vi "Interfaz grafica.vi"() -> ()   [LabVIEW 2016]
uses:
  Optotune Lens Driver 4 Labview package/Optotune Lens Driver 4 Labview package/Hello Optotune Lens (30.06.2015)/Calibration.ctl
  <vilib>/DAQmx/read.llb/DAQmx Read (Analog 1D Wfm NChan NSamp).vi
  <vilib>/Analysis/2dsp.llb/Decimate (single shot, DBL).vi
  <vilib>/Utility/file.llb/Read Delimited Spreadsheet (string).vi
  <vilib>/DAQmx/miscellaneous.llb/DAQmx Fill In Error Info.vi
  <vilib>/Waveform/WDTOps.llb/WDT Index Channel DBL.vi
  <vilib>/Analysis/2dsp.llb/Decimate (continuous, DBL).vi
  <vilib>/Instr/_visa.llb/VISA Configure Serial Port (Instr).vi
  <vilib>/Utility/file.llb/Write Delimited Spreadsheet (string).vi
  <vilib>/Waveform/WDTOps.llb/WDT Get Waveform Time Array DBL.vi
  <vilib>/Analysis/NI_AALPro.lvlib
panel:
  in  "Restablecer Iniciales":bool
  in  "Incremento":dbl=0.1 format="%#_13g"
  out "Potencia derecho":dbl
  out "error out 4":errorcluster
  out "error out 3":errorcluster
  out "error out 2":errorcluster
  in  "Tab Control 3":enum32{"WL", "Video"}(tab)
  out "Waveform length":dbl[][](graph)
  in  "Escala autom. X":u8=1
  in  "Maximo escala X":dbl
  in  "Minimo escala X":dbl
  in  "Minimo escala Y":dbl format="%#_13g"
  in  "Maximo escala Y":dbl format="%#_13g"
  in  "Escala autom. Y":u8=1
  out "Image Out":T1(plugin-control)
  in  "Carpeta archivo":string="C:\\Users\\TGM1603\\Documents\\LabVIEW Data\\Experimentos electrodos\\VideosExperimentos"
  in  "Modo de video":u16(ring)=21 items=["160x90 I420 30 fps", "160x90 MJPG 30 fps", "160x90 RGB24 30 fps", "160x120 I420 30 fps", "160x120 MJPG 30 fps", "160x120 RGB24 30 fps", "176x144 I420 30 fps", "176x144 MJPG 30 fps", "176x144 RGB24 30 fps", "320x180 I420 30 fps", "320x180 MJPG 30 fps", "320x180 RGB24 30 fps", "320x240  I420 30 fps", "320x240 MJPG 30 fps", "320x240 RGB24 30 fps", "352x288 I420 30 fps", "352x288 MJPG 30 fps", "352x288 RGB24 30 fps", "432x240 I420 30 fps", "432x240 MJPG 30 fps", "432x240 RGB24 30 fps", "640x360 I420 30 fps", "640x360 MJPG 30 fps", "640x360 RGB24 30 fps", "640x480 I420 30 fps", "640x480 MJPG 30 fps", "640x480 RGB24 30 fps", "800x448 I420 30 fps", "800x448 MJPG 30 fps", "800x448 RGB24 30 fps", "800x600 I420 30 fps", "800x600 MJPG 30 fps", "800x600 RGB24 30 fps", "864x480 I420 30 fps", "864x480 MJPG 30 fps", "864x480 RGB24 30 fps", "960x720 I420 30 fps", "960x720 MJPG 30 fps", "960x720 RGB24 30 fps", "1024x576 I420 30 fps", "1024x576 MJPG 30 fps", "1024x576 RGB24 30 fps", "1280x720 I420 30 fps", "1280x720 MJPG 30 fps", "1280x720 RGB24 30 fps", "1600x896 I420 30 fps", "1600x896 MJPG 30 fps", "1600x896 RGB24 30 fps", "1920x1080 I420 5 fps", "1920x1080 MJPG 30 fps", "1920x1080 RGB24 5 fps", "2304x1296 I420 2 fps", "2304x1296 RGB24 2 fps", "2304x1536 I420 2 fps", "2304x1536 RGB24 2 fps"]
  in  "Calidad":u32=1000
  in  "Frame Rate":u32=30
  out "VISA resource name out":string
  in  "Tab Control 2":T2(tab)
  in  "DAQmx Physical Channel":tag
  in  "Frecuencia muestreo":i32=20000
  in  "Rango voltaje":i16(ring)=5 items=["0.1"=0, "1"=1, "5"=5, "10"=10]
  in  "tamaño buffer":i32=1000
  in  "factor decimacion":i32=20
  in  "Ganancia":u16(ring) items=["0.2"=51455, "1"=33023, "10"=49407, "20"=41215, "30"=57599, "40"=37119, "60"=53503, "80"=45311, "120"=61695, "157"=35071, ""=0]
  in  "Potencia inicial lente derecho":dbl(slide) scale=-3.0..3.0
  in  "Potencia inicial lente izquierdo":dbl(slide) scale=-3.0..3.0
  in  "VISA resource name":string="COM11"
  in  "VISA resource name 2":string="COM10"
  out "DPT INICIALES D":dbl
  out "DPT INICIALES I":dbl
  out "Potencia izquierdo":dbl
  in  "error in (no error) 5":errorcluster
  in  "error in (no error) 4":errorcluster
  in  "error in (no error) 3":errorcluster
  in  "error in (no error) 2":errorcluster
  in  "Calibration 4":T3={"Max Current A"=293.0, "Max Current B"=293.0, "UCL A"=300.0, "UCL B"=300.0, "LCL A"=0.0, "LCL B"=0.0} {"Max Current A" format="%#_g mA"; "Max Current B" format="%#_g mA"; "UCL A" format="%#_g mA"; "LCL A" format="%#_g mA"; "UCL B" format="%#_g mA"; "LCL B" format="%#_g mA"}
  out "ID 2":u16
  out "VISA resource name out 2":string
  out "Calibration 3":T3 {"Max Current A" format="%#_g mA"; "Max Current B" format="%#_g mA"; "UCL A" format="%#_g mA"; "LCL A" format="%#_g mA"; "UCL B" format="%#_g mA"; "LCL B" format="%#_g mA"}
  out "OK 2":bool
  out "Data 2":string
  out "Command to Port 2":string
  in  "Cola tipo 2":dbl[](array[numeric])
  out "Distancia":u32
  in  "Tamaño ventana WL":i32=60
  in  "Limite inferior WL":dbl=25.0 format="%#_13g"
  in  "Limite superior WL":dbl=50.0
  out "number":u32
  in  "Calibration":T3={"Max Current A"=293.0, "Max Current B"=293.0, "UCL A"=300.0, "UCL B"=300.0, "LCL A"=0.0, "LCL B"=0.0} {"Max Current A" format="%#_g mA"; "Max Current B" format="%#_g mA"; "UCL A" format="%#_g mA"; "LCL A" format="%#_g mA"; "UCL B" format="%#_g mA"; "LCL B" format="%#_g mA"}
  out "ID":u16
  out "Calibration 2":T3 {"Max Current A" format="%#_g mA"; "Max Current B" format="%#_g mA"; "UCL A" format="%#_g mA"; "LCL A" format="%#_g mA"; "UCL B" format="%#_g mA"; "LCL B" format="%#_g mA"}
  out "OK":bool
  out "Data":string
  out "Command to Port":string
  in  "DPT dif.":dbl
  out "error out":errorcluster
  in  "error in (no error)":errorcluster
  in  "WL":dbl
  in  "Cola tipo":dbl[](array[numeric])
  out "T button?":bool
  in  "Elegir menu Exp":bool
  in  "Elegir menu":bool
  out "path":path
  in  "Iniciar experimento":bool
  in  "Parar adquisicion":bool
  out "Enfermedad visual":string
  out "Edad":string
  out "Nombre":string
  out "Cedula":string
  in  "Carpeta":path=path "C:/Users/TGM1603/Documents/LabVIEW Data/Experimentos electrodos"
  in  "?":bool
  in  "Menu Principal":u16(ring) items=["Visualizacion general ", "Llevar a cabo un experimento", "Ajustar potencia inicial lentes"]
  in  "Menu experimentos":u16(ring) items=["Experimento 1", "Experimento 2", "Experimento 3", "Experimento 4", "", "", "", ""]
  in  "Tab Control":enum32{"Señal EMG", "Potencia y distancia"}(tab)
  out "Senal EMG":waveform(dbl)[](graph)
  in  "Escala automatica Y":u8
  in  "Escala automatica X":u8=1
  in  "X Scale.Range:Increment":dbl
  in  "X Scale.Range:Minimum":dbl
  in  "X Scale.Range:Maximum":dbl
  in  "Y Scale.Range:Minimum":dbl=-5.0
  in  "Y Scale.Range:Maximum":dbl=5.0
  in  "Escala Y min":dbl
  in  "Escala Y max":dbl
  in  "Auto scale Y":u8=1
  in  "Escala X max":dbl
  in  "Escala X min":dbl
  out "Potencia optica y distancia":dbl[][](graph)
  in  "Auto scale X":u8=1
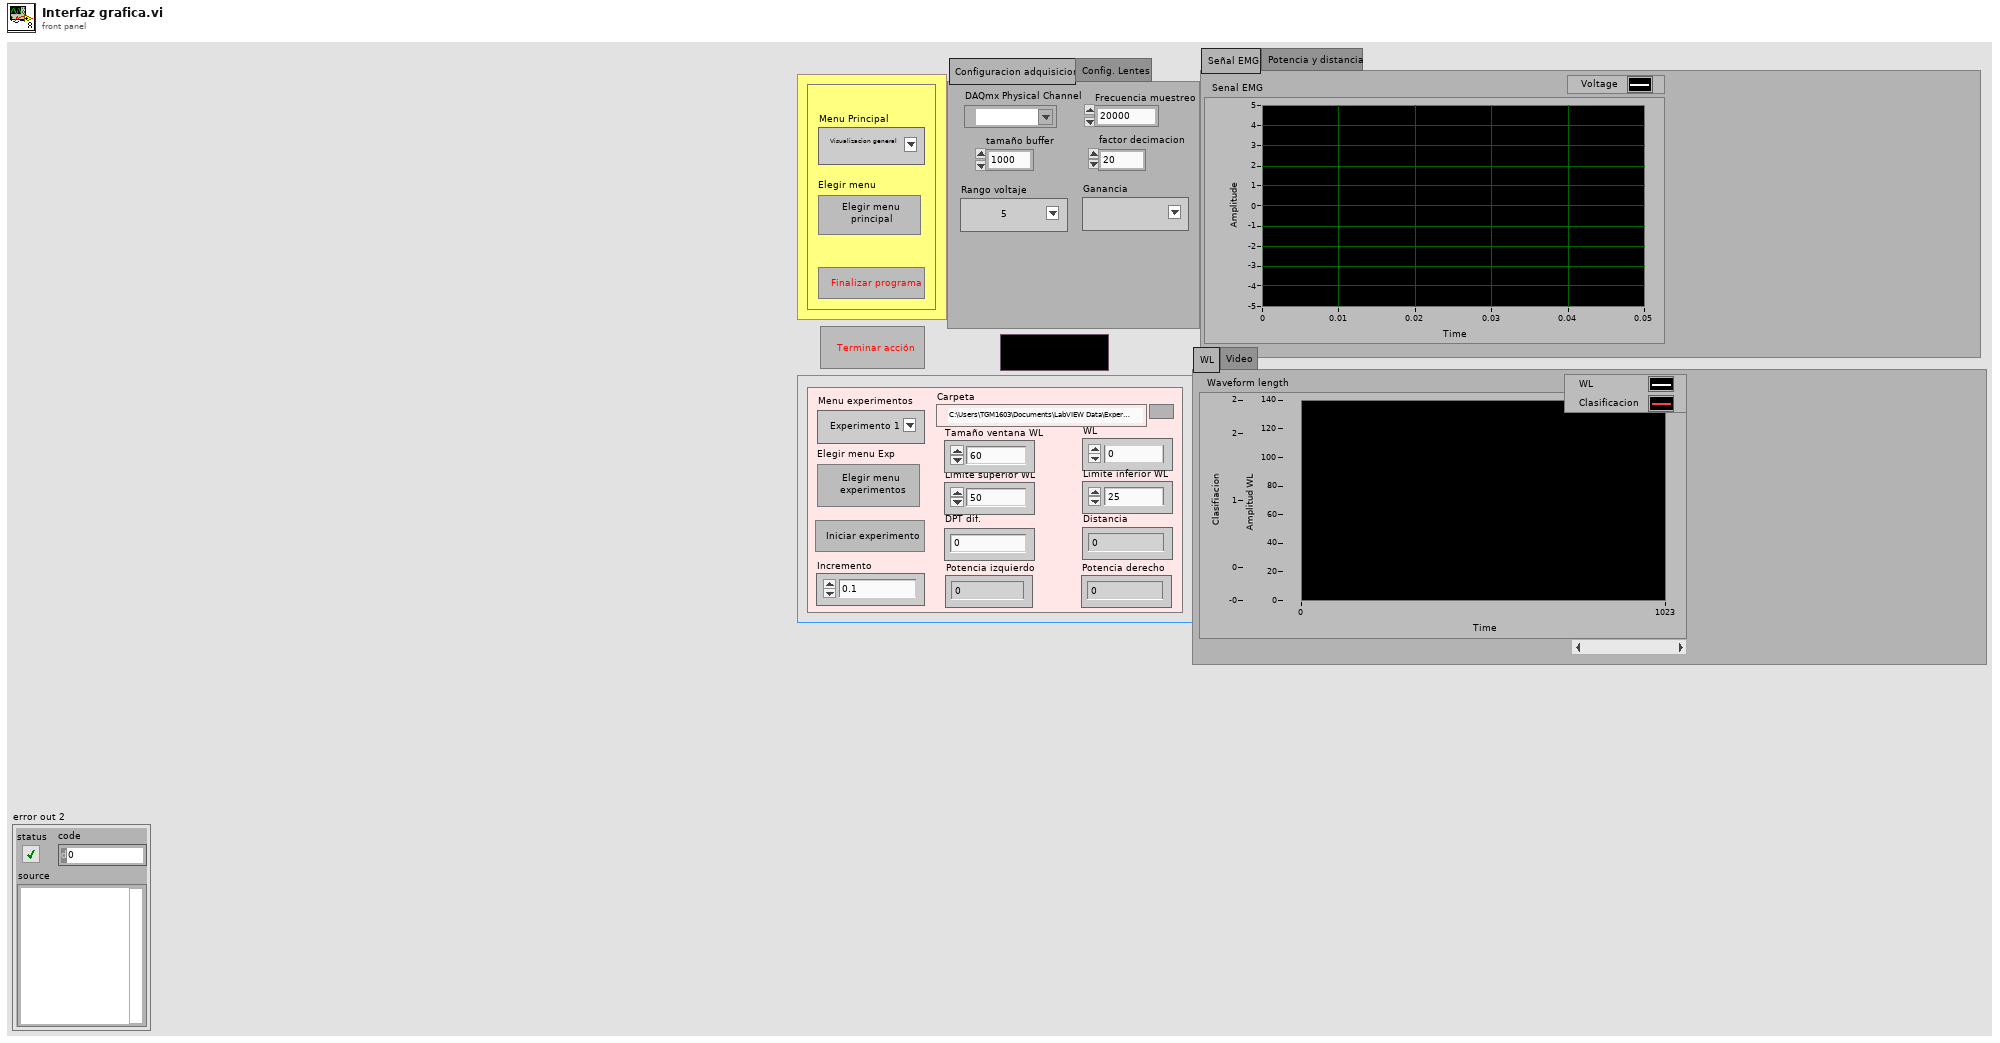
[diagram p1: front panel]
types:
  T1 = typedef "IMAQ Image.ctl" = refnum<image>
  T2 = enum32{"Configuracion adquisicion", "Config. Lentes"}
  T3 = typedef "Calibration.ctl" = cluster{"Max Current A":dbl, "Max Current B":dbl, "UCL A":dbl, "UCL B":dbl, "LCL A":dbl, "LCL B":dbl}
  T4 = enum16{"Left Button", "Center Button", "Right Button", "Window Close"}
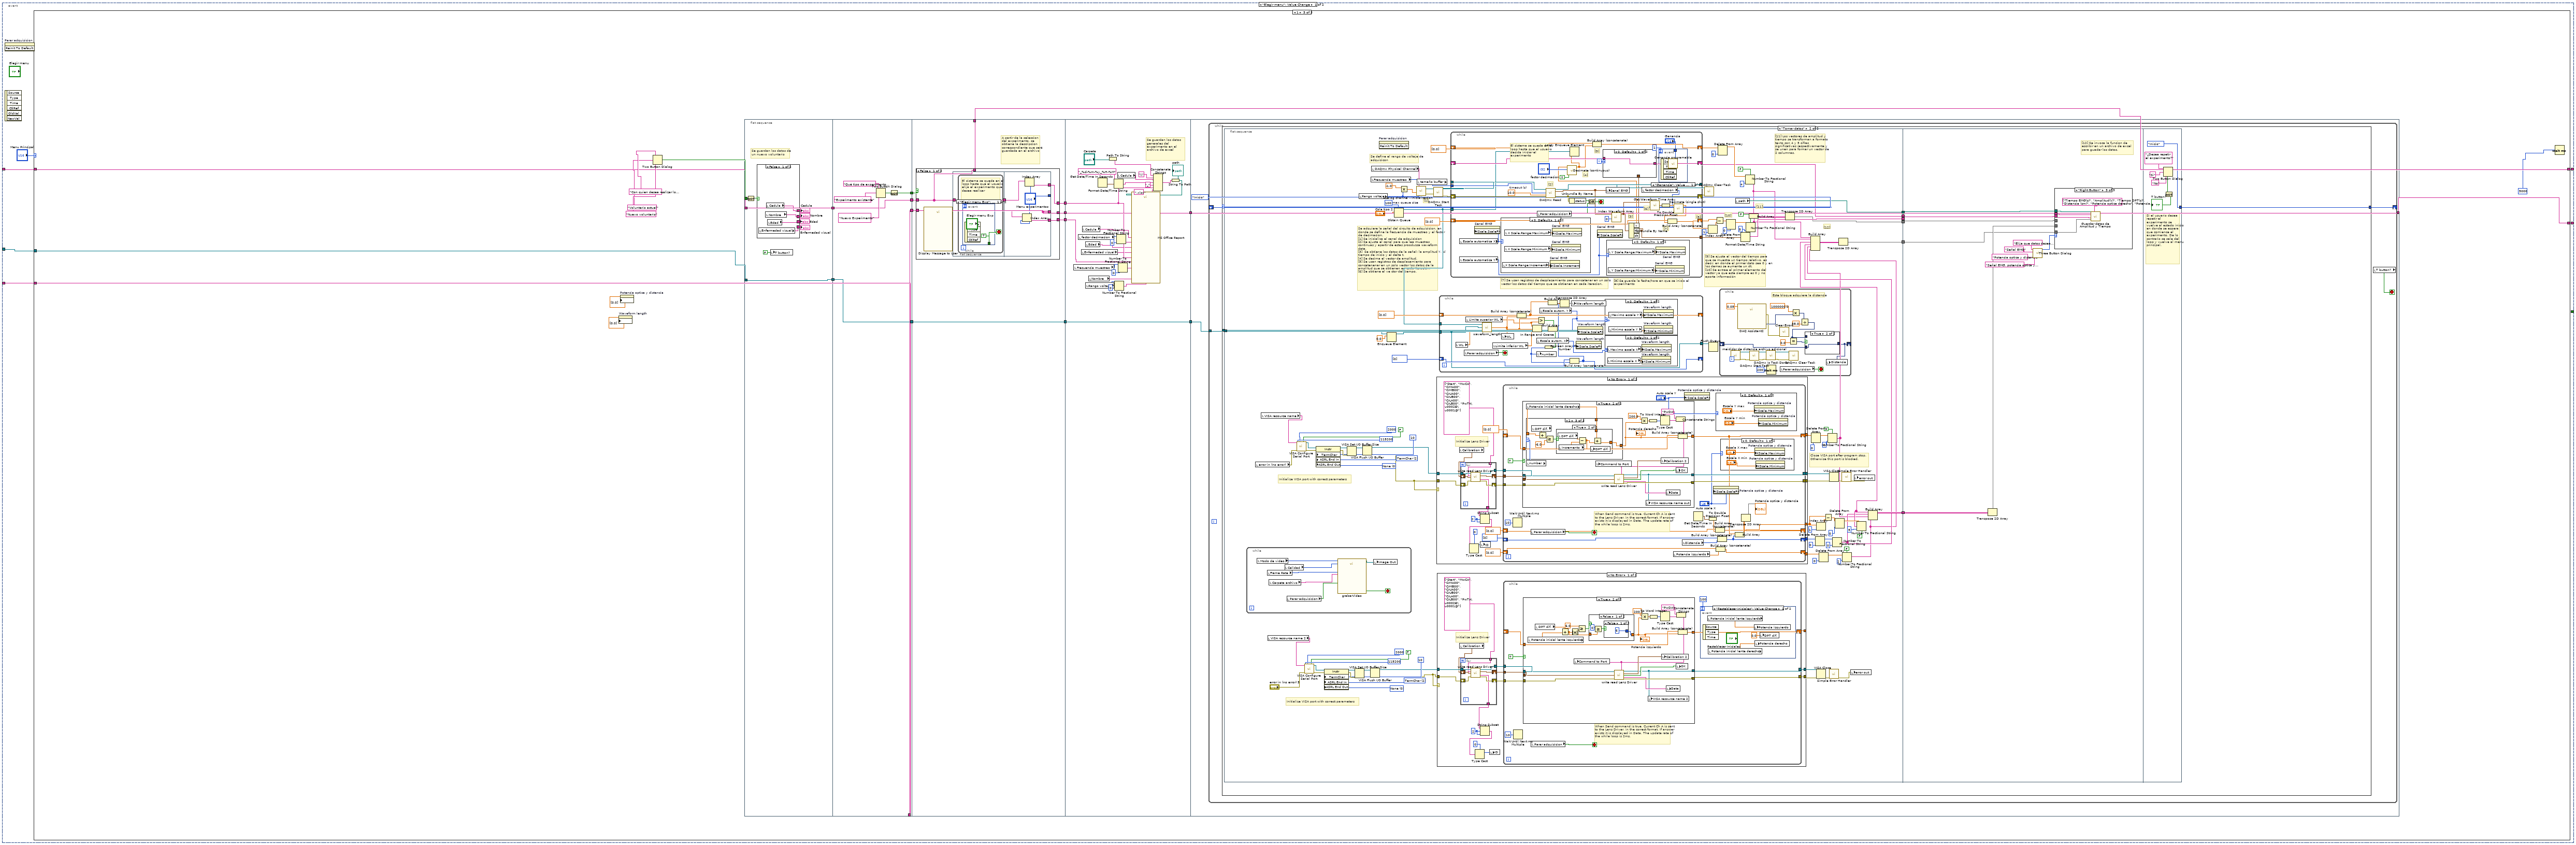
[diagram p2: hidden frame]
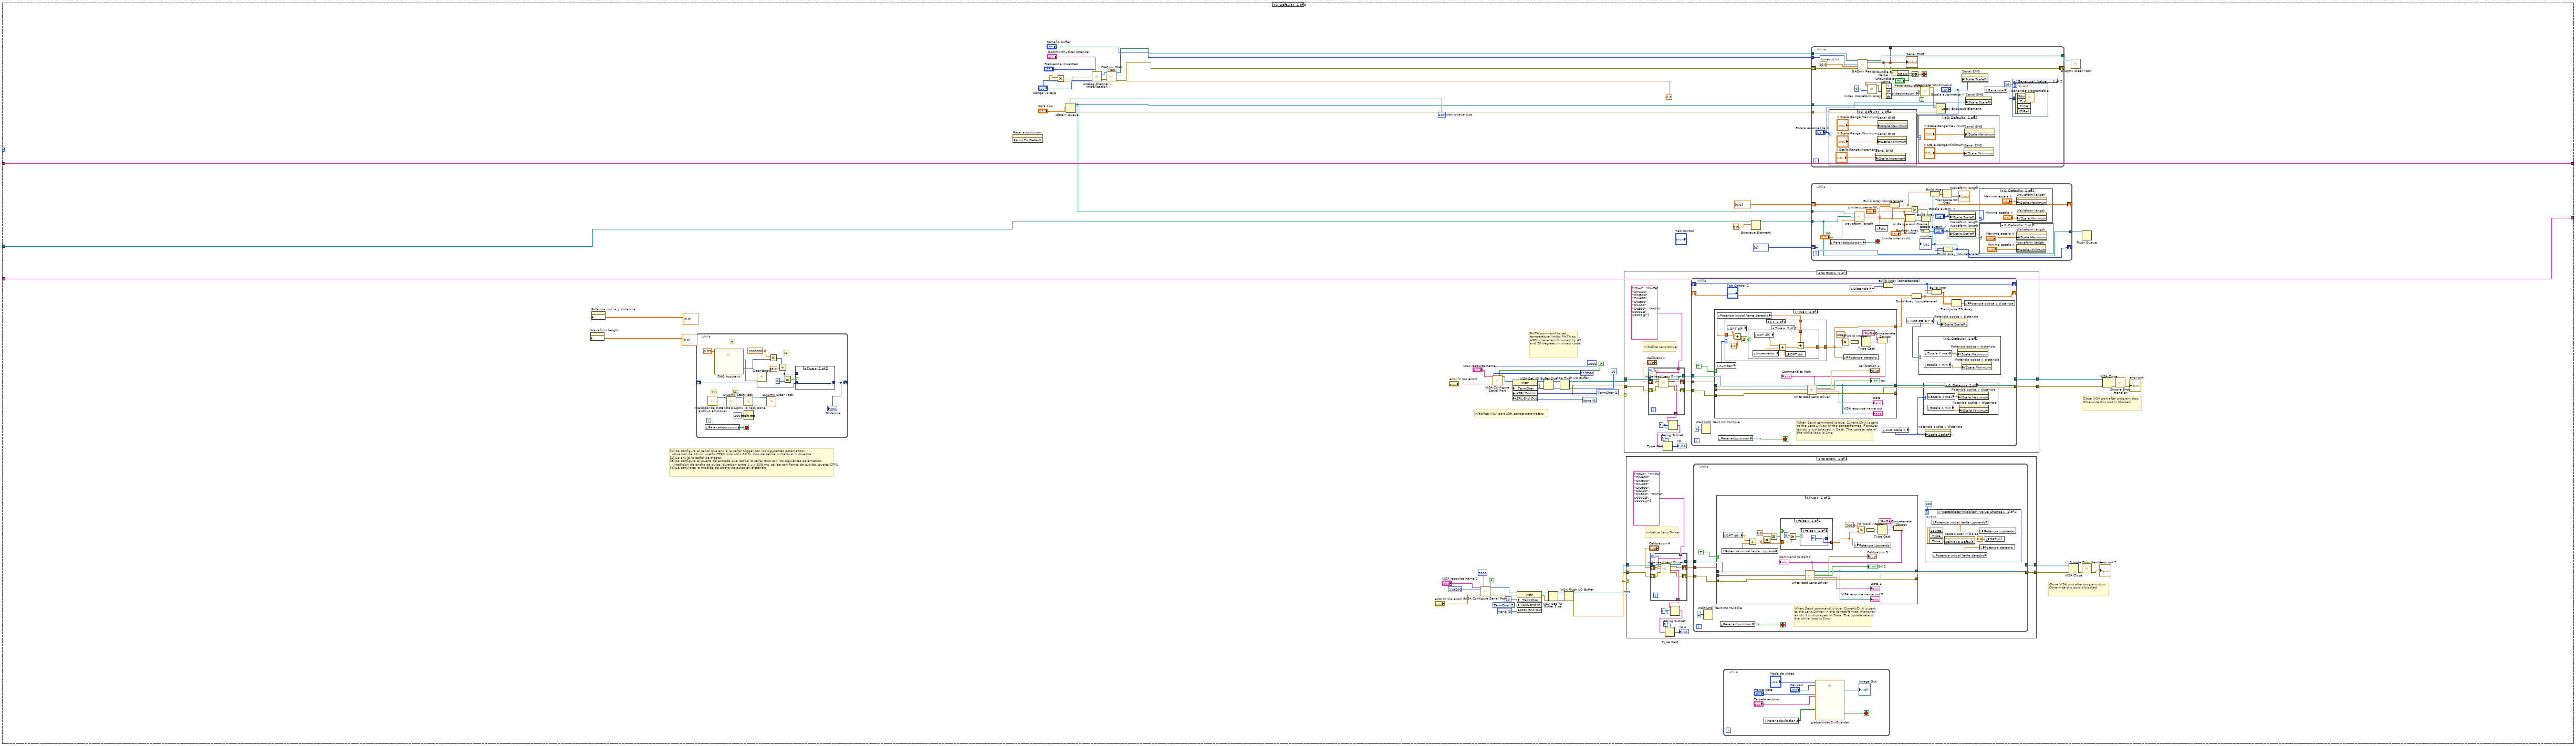
[diagram p3: hidden frame]
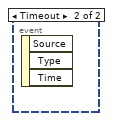
[diagram p4: hidden frame]
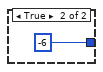
[diagram p6: hidden frame]
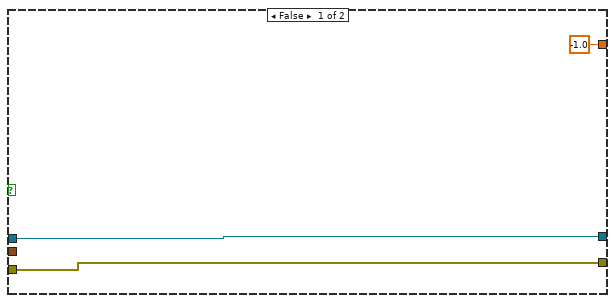
[diagram p12: hidden frame]
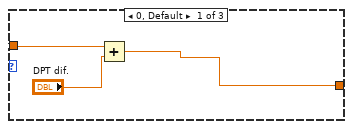
[diagram p13: hidden frame]
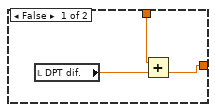
[diagram p14: hidden frame]
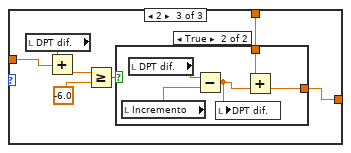
[diagram p15: hidden frame]
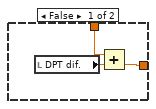
[diagram p16: hidden frame]
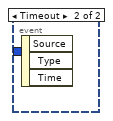
[diagram p20: hidden frame]
diagram:
  # "[1] Se configura el canal que envía la señal trigger con los siguientes parametros:\n  -duracion de 10 us, puerto CTR0,ciclo utilo 50 %, tipo de salida pulsatoria, 1 muestra \n[2] Se envía la señal de trigger.\n[3] Se configura el puerto de entrada que recibe la señal ECO con los siguientes parámetros:\n  - Medicion de ancho de pulso, duracion entre 1 u y 600 ms, se lee con flanco de subida, puerto CTR1\n[4] Se convierte la medida de ancho de pulso en distancia."
  n1 = flat-sequence {
    tunnel: [w18] -> w3
    tunnel: [w15] -> w2
    tunnel: [w10] -> w1
    tunnel: w3 -> [w24]
    tunnel: w2 -> [w23]
    tunnel: w1 -> [w22]
    frame #0 {
      # "Inicializa la cola"
      # "Crea la cola que va a guardar los valores de la sumatoria que calcula el waveform length así como determina la cantidad de valores que se van a sumar(tamaño de la ventana)"
      # "Se obtiene los elementos de la columna 1 que corresponde a  la descripcion de los experimentos"
      # "Se obtiene los elementos de la columna 0 que corresponde al nombre de los experimentos"
      # "Se guarda los experimentos en el menu\n para que el usuario pueda elegir cual \nrealizar"
      # "Se cargan los experimentos  guardados"
      n2 = call-poly <vilib>:"Read Delimited Spreadsheet.vi"("file path (dialog if empty)"=path "C:/Users/TGM1603/Documents/LabVIEW Data/Experimentos_realizados") -> ("all rows"=w19:string[][])  [unwired: 9 in, 5 out]
      n3 = Transpose 2D Array(2D array=w19) -> (transposed array=w16:string[][])
      n4 = Index Array(array=w16, index (row)=1) -> (element=w15:string[])  [unwired: 1 in]
      n5 = Index Array(array=w16, index (row)=0) -> (element=w18:string[])  [unwired: 1 in]
      n6 = property on="Menu experimentos" class="Ring (strict)"("Strings []"=w18) -> ()  [unwired: 2 in, 2 out]
      n7 = Obtain Queue(max queue size (-1, unlimited)="Tamaño ventana WL", element data type=0.0) -> (queue out=w13:refnum<queue>)  [unwired: 3 in, 2 out]
      n8 = property on="Waveform length" class="WFChart (strict)"("History Data"=dbl[][] [[0.0]]) -> ()  [unwired: 2 in, 2 out]
      n9 = property on="Potencia optica y distancia" class="WFChart (strict)"("History Data"=dbl[][] [[0.0]]) -> ()  [unwired: 2 in, 2 out]
      n10 = local write "DPT INICIALES D"(0.0 ("DPT INIT.1")) -> ()
      n11 = local write "DPT INICIALES I"(0.0 ("DPT INIT.2")) -> ()
      n12 = local write "DPT dif."(0.0 ("WL")) -> ()
      n13 = local write "WL"(0.0 ("WL")) -> ()
      n14 = Enqueue Element(queue=w13, element=0.0) -> (queue out=w10:refnum<queue>)  [unwired: 2 in, 2 out]
    }
    frame #1 {
      n15 = while {
        shift-right: [w30] -> _
        shift-left: w24 -> [w31]
        shift-right: [w28] -> _
        shift-left: w23 -> [w29]
        tunnel: w22 -> [w27]
        stop <- w26 stop-if-true
        n16 = event shown="[1] Timeout" {
          selector: _ -> [_ _]
          dyn-events: _ -> [_ _]
          timeout: 10 -> [_ _]
          tunnel: w31 -> [w37 w1048]
          tunnel: [w36 w1048] -> w30
          tunnel: w29 -> [w35 w1047]
          tunnel: [w34 w1047] -> w28
          tunnel: w27 -> [w32 _]
          tunnel: [_ "?"] -> w26
          event "Elegir menu": Value Change {
            n17 = invoke on="Parar adquisicion" class="Bool (strict)" method="Reinit To Default"() -> ()  [unwired: 3 in, 3 out]
            n18 = event-data() -> ()  [unwired: 1 in, 6 out]
            n19 = case shown="1" "Menu Principal" {
              tunnel: w37 -> [w103 w389 w504]
              tunnel: [w103 w389 w503] -> w36
              tunnel: w35 -> [w102 w388 w501]
              tunnel: [w102 w388 w500] -> w34
              tunnel: w32 -> [w85 _ w490]
              frame 0, Default {
                w53 = u16 0 items=["None", "Last Bit", "TermChar", "Break"] ("Serial Settings:End Mode for Writes")
                w52 = u16 2 items=["None", "Last Bit", "TermChar"] ("Serial Settings:End Mode for Reads")
                w75 = u16 0 items=["None", "Last Bit", "TermChar", "Break"] ("Serial Settings:End Mode for Writes")
                w76 = u16 2 items=["None", "Last Bit", "TermChar"] ("Serial Settings:End Mode for Reads")
                w89 = 100  # max queue size
                # "Close VISA port after program stop. Otherwise this port is blocked."
                # "[1] Se configura el canal que envía la señal trigger con los siguientes parametros:\n  -duracion de 10 us, puerto CTR0,ciclo utilo 50 %, tipo de salida pulsatoria, 1 muestra \n[2] Se envía la señal de trigger.\n[3] Se configura el puerto de entrada que recibe la señal ECO con los siguientes parámetros:\n  - Medicion de ancho de pulso, duracion entre 1 u y 600 ms, se lee con flanco de subida, puerto CTR1\n[4] Se convierte la medida de ancho de pulso en distancia."
                # "PwTA command to set temperature limits: PwTA as ASCII characters followed by 45 and 20 degrees in binary code."
                # "Close VISA port after program stop. Otherwise this port is blocked."
                # "Initialize VISA port with correct parameters"
                n20 = property on="Waveform length" class="WFChart (strict)"("History Data"=dbl[][] [[0.0]]) -> ()  [unwired: 2 in, 2 out]
                n21 = property on="Potencia optica y distancia" class="WFChart (strict)"("History Data"=dbl[][] [[0.0]]) -> ()  [unwired: 2 in, 2 out]
                n22 = while {
                  shift-right: [w178] -> _
                  shift-left: _ -> [w177]
                  stop <- w182 stop-if-true
                  # "[4]"
                  # "[3]"
                  # "[2]"
                  # "[1]"
                  n23 = local read "Parar adquisicion"() -> (w182:bool)
                  n24 = call "meididor de distancia archivo adicional.vi"() -> ("error out"=w185:errorcluster, "task out"=w186:refnum<k21>)  [unwired: 10 in]
                  n25 = call "DAQ Assistant"("timeout (s)"=0.05) -> ("data"=w195:dynamicdata, "error out"=w183:errorcluster)  [unwired: 16 in, 1 out]
                  n26 = call <vilib>:"DAQmx Start Task.vi"("task/channels in"=w186, "error in"=w185) -> ("task out"=w189:refnum<k21>, "error out"=w190:errorcluster)  [unwired: 12 in]
                  n27 = call <vilib>:"DAQmx Is Task Done.vi"("task/channels in"=w189, "error in"=w190) -> ("task out"=w187:refnum<k21>, "error out"=w188:errorcluster)  [unwired: 11 in, 1 out]
                  n28 = Wait (ms)(milliseconds to wait=u32 200) -> ()  [unwired: 1 out]
                  n29 = call <vilib>:"Clear Errors.vi"("error in (no error)"=w183) -> ()  [unwired: 5 in, 2 out]
                  n30 = call <vilib>:"DAQmx Clear Task.vi"("task in"=w187, "error in"=w188) -> ()  [unwired: 13 in, 1 out]
                  n31 = Multiply(x=1000000.0, y=w195) -> (x*y=w193:dynamicdata)
                  n32 = Divide(x=w193, y=58.0) -> (x/y=w179:dynamicdata)
                  n33 = Equal?(x=w179, y=u16 0) -> (x = y?=w181:dynamicdata)
                  n34 = case shown="True" w181 {
                    tunnel: [w196 w197] -> w178
                    tunnel: w179 -> [w196 _]
                    tunnel: w177 -> [_ w197]
                    frame False {
                    }
                    frame True {
                    }
                  }
                  "Distancia" <- w178
                }
                n35 = invoke on="Parar adquisicion" class="Bool (strict)" method="Reinit To Default"() -> ()  [unwired: 3 in, 3 out]
                n36 = Multiply(x=-1.0 ("y"), y="Rango voltaje") -> (x*y=w92:dbl)
                n37 = Obtain Queue(max queue size (-1, unlimited)=w89, element data type="Cola tipo") -> (queue out=w86:refnum<queue>, error out=w87:errorcluster)  [unwired: 3 in, 1 out]
                n38 = call "Analog channel - inicializacion.vi"("maximum value"="Rango voltaje", "minimum value"=w92, "rate"="Frecuencia muestreo", "DAQmx Physical Channel"="DAQmx Physical Channel") -> ("error out"=w95:errorcluster, "task out"=w96:refnum<k21>)
                n39 = call <vilib>:"DAQmx Start Task.vi"("task/channels in"=w96, "error in"=w95) -> ("task out"=w101:refnum<k21>, "error out"=w100:errorcluster)  [unwired: 12 in]
                n40 = call-poly "VISA Configure Serial Port"("VISA resource name"="VISA resource name 2", "timeout (10sec)"=u32 2000, "Enable Termination\nChar (T)"=FALSE ("Enable Termination\nChar (T)"), "baud rate (9600)"=u32 115200, "error in (no error)"="error in (no error) 2") -> ("VISA resource name out"=w48:refnum<visa-resource-name>, "error out"=w50:errorcluster)  [unwired: 9 in]
                n41 = call-poly "VISA Configure Serial Port"("VISA resource name"="VISA resource name", "timeout (10sec)"=u32 2000, "Enable Termination\nChar (T)"=FALSE ("Enable Termination\nChar (T)"), "baud rate (9600)"=u32 115200, "error in (no error)"="error in (no error)") -> ("VISA resource name out"=w80:refnum<visa-resource-name>, "error out"=w78:errorcluster)  [unwired: 9 in]
                n42 = property class="Instr"(reference=w80, error in=w78, "TermChar"=u8 10 ("Message Based Settings:Termination Character"), "ASRL End In"=w76, "ASRL End Out"=w75) -> (reference out=w79:refnum<visa-resource-name>, error out=w77:errorcluster)
                n43 = property class="Instr"(reference=w48, error in=w50, "TermChar"=u8 10 ("Message Based Settings:Termination Character"), "ASRL End In"=w52, "ASRL End Out"=w53) -> (reference out=w49:refnum<visa-resource-name>, error out=w51:errorcluster)
                n44 = VISA Set I/O Buffer Size(VISA resource name=w79, error in (no error)=w77) -> (VISA resource name out=w72:refnum<visa-resource-name>, error out=w71:errorcluster)  [unwired: 2 in]
                n45 = VISA Set I/O Buffer Size(VISA resource name=w49, error in (no error)=w51) -> (VISA resource name out=w56:refnum<visa-resource-name>, error out=w57:errorcluster)  [unwired: 2 in]
                n46 = VISA Flush I/O Buffer(VISA resource name=w72, error in (no error)=w71) -> (VISA resource name out=w70:refnum<visa-resource-name>, error out=w65:errorcluster)  [unwired: 1 in]
                n47 = VISA Flush I/O Buffer(VISA resource name=w56, error in (no error)=w57) -> (VISA resource name out=w42:refnum<visa-resource-name>, error out=w43:errorcluster)  [unwired: 1 in]
                n48 = case shown="No Error" w65 {
                  tunnel: w65 -> [w211 w295]
                  tunnel: w70 -> [w210 w296]
                  tunnel: [w209 w295] -> w68
                  tunnel: [w208 w296] -> w66
                  frame No Error {
                    w206 = 2 ("length (rest)")
                    # "Initialize Lens Driver"
                    n49 = for {
                      tunnel: w210 -> [w293]
                      tunnel: [w290] -> w200
                      tunnel: string[] ["Start", "MwCA", "CrMA00", "CrMB00", "CrUA00", "CrUB00", "CrLA00", "CrLB00", "PwTA\u0002Ð\u0001@"] -> [w288] mode=indexing
                      tunnel: [w287] -> w199
                      shift-right: [w291] -> w201
                      shift-left: "Calibration" -> [w292]
                      shift-right: [w289] -> w202
                      shift-left: w211 -> [w294]
                      n50 = call "write read Lens Driver.vi"("VISA resource name"=w293, "command"=w288, "Calibration"=w292, "error in (no error)"=w294) -> ("VISA resource name out"=w290:refnum<visa-resource-name>, "Calibration 2"=w291:T3, "Data"=w287:string, "error out"=w289:errorcluster)  [unwired: 4 in, 4 out]
                    }
                    n51 = String Subset(string=w199, offset (0)=w206, length (rest)=w206) -> (substring=w204:string)
                    n52 = Type Cast(type=u16 0 ("length (rest)"), x=w204) -> (*(type *) &x=→"ID":u16)
                    n53 = while {
                      tunnel: [w223] -> w209
                      tunnel: [w224] -> w208
                      tunnel: w202 -> [w229]
                      tunnel: w201 -> [w228]
                      tunnel: w200 -> [w227]
                      shift-right: [w214] -> _
                      shift-left: _ -> [w218]
                      shift-right: [w215] -> _
                      shift-left: _ -> [w217]
                      stop <- w222 stop-if-true
                      # "When Send command is true, Current Ch A is sent to the Lens Driver, in the correct format. If answer exists it is displayed in Data. The update rate of the while loop is 2ms."
                      n54 = Wait Until Next ms Multiple(millisecond multiple=u32 2) -> ()  [unwired: 1 out]
                      n55 = case shown="True" TRUE ("Send command") {
                        tunnel: [w236 w253] -> w223
                        tunnel: w229 -> [w236 w252]
                        tunnel: w228 -> [_ w246]
                        tunnel: w227 -> [w235 w251]
                        tunnel: [w235 w248] -> w224
                        tunnel: [-1.0 ("DPT") w237] -> w216
                        frame False {
                        }
                        frame True {
                          n56 = local read "number"() -> (w239:u32)
                          n57 = local read "Potencia inicial lente derecho"() -> (w238:dbl)
                          n58 = case shown="1" w239 {
                            tunnel: [w255 w263 w278] -> w237
                            tunnel: w238 -> [w256 w258 w273]
                            tunnel: w238 -> [_ w257 w272]
                            frame 0, Default {
                              n59 = Add(x=w256, y="DPT dif.") -> (x+y=w255:dbl)
                            }
                            frame 1 {
                              n60 = local read "DPT dif."() -> (w259:dbl)
                              n61 = Add(x=w258, y=w259) -> (x+y=w260:dbl)
                              n62 = Less Or Equal?(x=w260, y=6.0) -> (x <= y?=w262:bool)
                              n63 = case shown="True" w262 {
                                tunnel: [w265 w269] -> w263
                                tunnel: w257 -> [w264 w268]
                                frame False {
                                n64 = local read "DPT dif."() -> (w266:dbl)
                                n65 = Add(x=w264, y=w266) -> (x+y=w265:dbl)
                                }
                                frame True {
                                n66 = local read "Incremento"() -> (w267:dbl)
                                n67 = local read "DPT dif."() -> (w270:dbl)
                                n68 = Add(x=w270, y=w267) -> (x+y=w271:dbl)
                                n69 = local write "DPT dif."(w271) -> ()
                                n70 = Add(x=w268, y=w271) -> (x+y=w269:dbl)
                                }
                              }
                            }
                            frame 2 {
                              n71 = local read "DPT dif."() -> (w277:dbl)
                              n72 = Add(x=w277, y=w273) -> (x+y=w274:dbl)
                              n73 = Greater Or Equal?(x=w274, y=-6.0) -> (x >= y?=w275:bool)
                              n74 = case shown="True" w275 {
                                tunnel: [w280 w284] -> w278
                                tunnel: w272 -> [w279 w283]
                                frame False {
                                n75 = local read "DPT dif."() -> (w281:dbl)
                                n76 = Add(x=w279, y=w281) -> (x+y=w280:dbl)
                                }
                                frame True {
                                n77 = local read "Incremento"() -> (w282:dbl)
                                n78 = local read "DPT dif."() -> (w286:dbl)
                                n79 = Subtract(x=w286, y=w282) -> (x-y=w285:dbl)
                                n80 = local write "DPT dif."(w285) -> ()
                                n81 = Add(x=w283, y=w285) -> (x+y=w284:dbl)
                                }
                              }
                            }
                          }
                          n82 = Multiply(x=200.0, y=w237) -> (x*y=w244:dbl)
                          n83 = local write "Potencia derecho"(w237) -> ()
                          n84 = To Word Integer(number=w244) -> (16bit integer=w243:i16)
                          n85 = Type Cast(x=w243) -> (*(type *) &x=w242:string)  [unwired: 1 in]
                          n86 = Concatenate Strings("PwDA", w242) -> (w240:string)
                          "Command to Port" <- w240
                          n87 = call "write read Lens Driver.vi"("VISA resource name"=w251, "command"=w240, "Calibration"=w246, "error in (no error)"=w252) -> ("VISA resource name out"=w248:refnum<visa-resource-name>, "Calibration 2"=→"Calibration 2":T3, "OK"=→"OK":bool, "Data"=→"Data":string, "error out"=w253:errorcluster)  [unwired: 4 in, 3 out]
                          "VISA resource name out" <- w248
                        }
                      }
                      n88 = local read "Parar adquisicion"() -> (w222:bool)
                      n89 = local read "Distancia"() -> (w219:u32)
                      n90 = local read "Auto scale X"() -> (w220:u8)
                      n91 = Build Array (concatenate)(w218, w219) -> (w214:u32[])
                      n92 = local read "Auto scale Y"() -> (w221:u8)
                      n93 = Build Array (concatenate)(w217, w216) -> (w215:dbl[])
                      n94 = case shown="0, Default" w221 {
                        frame 0, Default {
                          n95 = local read "Escala Y min"() -> (w232:dbl)
                          n96 = local read "Escala Y max"() -> (w233:dbl)
                          n97 = property on="Potencia optica y distancia" class="WFChart (strict)"("YScale.Maximum"=w233) -> ()  [unwired: 2 in, 2 out]
                          n98 = property on="Potencia optica y distancia" class="WFChart (strict)"("YScale.Minimum"=w232) -> ()  [unwired: 2 in, 2 out]
                        }
                        frame 1 {
                        }
                      }
                      n99 = case shown="0, Default" w220 {
                        frame 0, Default {
                          n100 = local read "Escala X min"() -> (w230:dbl)
                          n101 = local read "Escala X max"() -> (w231:dbl)
                          n102 = property on="Potencia optica y distancia" class="WFChart (strict)"("XScale.Maximum"=w231) -> ()  [unwired: 2 in, 2 out]
                          n103 = property on="Potencia optica y distancia" class="WFChart (strict)"("XScale.Minimum"=w230) -> ()  [unwired: 2 in, 2 out]
                        }
                        frame 1 {
                        }
                      }
                      n104 = property on="Potencia optica y distancia" class="WFChart (strict)"("XScale.ScaleFit"=w220) -> ()  [unwired: 2 in, 2 out]
                      n105 = Build Array(w215, w214) -> (w213:dbl[][])
                      n106 = property on="Potencia optica y distancia" class="WFChart (strict)"("YScale.ScaleFit"=w221) -> ()  [unwired: 2 in, 2 out]
                      n107 = Transpose 2D Array(2D array=w213) -> (transposed array=w212:dbl[][])
                      n108 = local write "Potencia optica y distancia"(w212) -> ()
                    }
                  }
                  frame Error {
                  }
                }
                n109 = case shown="No Error" w43 {
                  tunnel: w43 -> [w124 w175]
                  tunnel: w42 -> [w123 w176]
                  tunnel: [w122 w175] -> w38
                  tunnel: [w121 w176] -> w39
                  frame No Error {
                    w119 = 2 ("length (rest)")
                    # "Initialize Lens Driver"
                    n110 = for {
                      tunnel: w123 -> [w173]
                      tunnel: [w170] -> w113
                      tunnel: string[] ["Start", "MwCA", "CrMA00", "CrMB00", "CrUA00", "CrUB00", "CrLA00", "CrLB00", "PwTA\u0002Ð\u0001@"] -> [w168] mode=indexing
                      tunnel: [w167] -> w112
                      shift-right: [w171] -> w114
                      shift-left: "Calibration 4" -> [w172]
                      shift-right: [w169] -> w115
                      shift-left: w124 -> [w174]
                      n111 = call "write read Lens Driver.vi"("VISA resource name"=w173, "command"=w168, "Calibration"=w172, "error in (no error)"=w174) -> ("VISA resource name out"=w170:refnum<visa-resource-name>, "Calibration 2"=w171:T3, "Data"=w167:string, "error out"=w169:errorcluster)  [unwired: 4 in, 4 out]
                    }
                    n112 = String Subset(string=w112, offset (0)=w119, length (rest)=w119) -> (substring=w117:string)
                    n113 = Type Cast(type=u16 0 ("length (rest)"), x=w117) -> (*(type *) &x=→"ID 2":u16)
                    n114 = while {
                      tunnel: [w127] -> w122
                      tunnel: [w128] -> w121
                      tunnel: w115 -> [w133]
                      tunnel: w114 -> [w132]
                      tunnel: w113 -> [w131]
                      stop <- w126 stop-if-true
                      # "When Send command is true, Current Ch A is sent to the Lens Driver, in the correct format. If answer exists it is displayed in Data. The update rate of the while loop is 2ms."
                      n115 = Wait Until Next ms Multiple(millisecond multiple=u32 2) -> ()  [unwired: 1 out]
                      n116 = case shown="True" TRUE ("Send command") {
                        tunnel: [w138 w159] -> w127
                        tunnel: w133 -> [w138 w158]
                        tunnel: w132 -> [_ w152]
                        tunnel: w131 -> [w137 w157]
                        tunnel: [w137 w154] -> w128
                        frame False {
                        }
                        frame True {
                          n117 = local read "Potencia inicial lente izquierdo"() -> (w144:dbl)
                          n118 = local read "DPT dif."() -> (w145:dbl)
                          n119 = Add(x=w145, y=w144) -> (x+y=w140:dbl)
                          n120 = Absolute Value(x=w140) -> (abs(x)=w142:dbl)
                          n121 = Greater Or Equal?(x=6.0, y=w142) -> (x >= y?=w143:bool)
                          n122 = case shown="False" w143 {
                            tunnel: w140 -> [w162 w166]
                            tunnel: [w160 w166] -> w139
                            frame False {
                              n123 = Greater Or Equal?(x=u16 0, y=w162) -> (x >= y?=w163:bool)
                              n124 = case shown="False" w163 {
                                tunnel: [i16 6 ("x") i16 -6 ("x")] -> w160
                                frame False {
                                }
                                frame True {
                                }
                              }
                            }
                            frame True {
                            }
                          }
                          n125 = local write "Potencia izquierdo"(w139) -> ()
                          n126 = Multiply(x=200.0, y=w139) -> (x*y=w150:dbl)
                          n127 = To Word Integer(number=w150) -> (16bit integer=w149:i16)
                          n128 = Type Cast(x=w149) -> (*(type *) &x=w148:string)  [unwired: 1 in]
                          n129 = Concatenate Strings("PwDA", w148) -> (w146:string)
                          "Command to Port 2" <- w146
                          n130 = call "write read Lens Driver.vi"("VISA resource name"=w157, "command"=w146, "Calibration"=w152, "error in (no error)"=w158) -> ("VISA resource name out"=w154:refnum<visa-resource-name>, "Calibration 2"=→"Calibration 3":T3, "OK"=→"OK 2":bool, "Data"=→"Data 2":string, "error out"=w159:errorcluster)  [unwired: 4 in, 3 out]
                          "VISA resource name out 2" <- w154
                        }
                      }
                      n131 = local read "Parar adquisicion"() -> (w126:bool)
                      n132 = event shown="[0] \"Restablecer Iniciales\": Value Change" {
                        selector: _ -> [_ _]
                        dyn-events: _ -> [_ _]
                        timeout: 100 -> [_ _]
                        event "Restablecer Iniciales": Value Change {
                          n133 = event-data() -> ()  [unwired: 1 in, 3 out]
                          n134 = local read "Potencia inicial lente izquierdo"() -> (w134:dbl)
                          n135 = local read "Potencia inicial lente derecho"() -> (w135:dbl)
                          n136 = invoke on="Restablecer Iniciales" class="Bool" method="Reinit To Default"() -> ()  [unwired: 3 in, 3 out]
                          n137 = local write "Potencia izquierdo"(w134) -> ()
                          n138 = local write "Potencia derecho"(w135) -> ()
                          n139 = local write "DPT dif."(0.0 ("DPT dif.")) -> ()
                        }
                        event Timeout {
                          n140 = event-data() -> ()  [unwired: 1 in, 3 out]
                        }
                      }
                    }
                  }
                  frame Error {
                  }
                }
                n141 = while {
                  stop <- w109 stop-if-true
                  n142 = local read "Parar adquisicion"() -> (w104:bool)
                  n143 = call "grabarVideoSinGuardar.vi"("VideoMode"="Modo de video", "Quality"="Calidad", "Stop (F)"=w104, "Image Logging Path"="Carpeta archivo", "Frame Rate"="Frame Rate") -> ("Image Out"=→"Image Out":T1, "Stopped"=w109:bool)  [unwired: 20 in, 1 out]
                }
                n144 = Enqueue Element(queue=w85, element=0.0) -> (queue out=w62:refnum<queue>)  [unwired: 2 in, 2 out]
                n145 = while {
                  tunnel: w62 -> [w298]
                  tunnel: w86 -> [w315]
                  shift-right: [w301] -> _
                  shift-left: dbl[] [0.0] -> [w312]
                  shift-right: [w300] -> _
                  shift-left: u32[] [0] -> [w302]
                  tunnel: [w298] -> w60
                  stop <- w313 stop-if-true
                  n146 = local read "Parar adquisicion"() -> (w313:bool)
                  n147 = call "waveform_length.vi"("WL"="WL", "Cola WL"=w298, "Datos entrada"=w315) -> ("WL 2"=w310:dbl)
                  n148 = local write "WL"(w310) -> ()
                  n149 = Build Array (concatenate)(w312, w310) -> (w301:dbl[])
                  n150 = In Range and Coerce(upper limit="Limite superior WL", x=w310, lower limit="Limite inferior WL") -> (In Range?=w308:bool)  [unwired: 1 out]
                  n151 = Greater?(x=w310, y="Limite superior WL") -> (0:w309:bool)
                  n152 = Build Array(w309, w308) -> (w307:bool[])
                  n153 = Boolean Array To Number(Boolean array=w307) -> (number=w303:u32)
                  "number" <- w303
                  n154 = Build Array (concatenate)(w302, w303) -> (w300:u32[])
                  n155 = Build Array(w301, w300) -> (w299:dbl[][])
                  n156 = Transpose 2D Array(2D array=w299) -> (transposed array=→"Waveform length":dbl[][])
                  n157 = property on="Waveform length" class="WFChart (strict)"("YScale.ScaleFit"="Escala autom. Y") -> ()  [unwired: 2 in, 2 out]
                  n158 = property on="Waveform length" class="WFChart (strict)"("XScale.ScaleFit"="Escala autom. X") -> ()  [unwired: 2 in, 2 out]
                  n159 = case shown="0, Default" "Escala autom. Y" {
                    frame 0, Default {
                      n160 = property on="Waveform length" class="WFChart (strict)"("YScale.Maximum"="Maximo escala Y") -> ()  [unwired: 2 in, 2 out]
                      n161 = property on="Waveform length" class="WFChart (strict)"("YScale.Minimum"="Minimo escala Y") -> ()  [unwired: 2 in, 2 out]
                    }
                    frame 1 {
                    }
                  }
                  n162 = case shown="0, Default" "Escala autom. X" {
                    frame 0, Default {
                      n163 = property on="Waveform length" class="WFChart (strict)"("XScale.Maximum"="Maximo escala X") -> ()  [unwired: 2 in, 2 out]
                      n164 = property on="Waveform length" class="WFChart (strict)"("XScale.Minimum"="Minimo escala X") -> ()  [unwired: 2 in, 2 out]
                    }
                    frame 1 {
                    }
                  }
                }
                n165 = while {
                  tunnel: w101 -> [w341]
                  tunnel: "tamaño buffer" -> [w338]
                  tunnel: [w339] -> w97
                  shift-right: [w336] -> w98
                  shift-left: w100 -> [w340]
                  tunnel: [w330] -> _
                  tunnel: w86 -> [w326]
                  tunnel: w87 -> [w325]
                  stop <- w335 stop-if-true
                  w334 = 10.0  # timeout (s)
                  n166 = case shown="0, Default" "Escala automatica X" {
                    frame 0, Default {
                      n167 = property on="Senal EMG" class="WFGraph (strict)"("XScale.Increment"="X Scale.Range:Increment") -> ()  [unwired: 2 in, 2 out]
                      n168 = property on="Senal EMG" class="WFGraph (strict)"("XScale.Minimum"="X Scale.Range:Minimum") -> ()  [unwired: 2 in, 2 out]
                      n169 = property on="Senal EMG" class="WFGraph (strict)"("XScale.Maximum"="X Scale.Range:Maximum") -> ()  [unwired: 2 in, 2 out]
                    }
                    frame 1 {
                    }
                  }
                  n170 = call-poly <vilib>:"DAQmx Read.vi"("task/channels in"=w341, "number of samples per channel"=w338, "timeout"=w334, "error in"=w340) -> ("task out"=w339:refnum<k21>, "data"=w330:waveform(dbl)[], "error out"=w336:errorcluster)  [unwired: 9 in]
                  "Senal EMG" <- w330
                  n171 = call-poly <vilib>:"Index Waveform Array.vi"("index"=0, "waveform array"=w330) -> ("waveform"=w331:waveform(dbl))  [unwired: 8 in, 1 out]
                  n172 = Unbundle By Name(w331) -> ("Y"=w328:dbl[])  [unwired: 2 out]
                  n173 = local read "factor decimacion"() -> (w327:i32)
                  n174 = Unbundle By Name(w336) -> ("status"=w337:bool)
                  n175 = Or(x=w337, y="Parar adquisicion") -> (x .or. y?=w335:bool)
                  n176 = case shown="0, Default" "Escala automatica Y" {
                    frame 0, Default {
                      n177 = property on="Senal EMG" class="WFGraph (strict)"("YScale.Minimum"="Y Scale.Range:Minimum") -> ()  [unwired: 2 in, 2 out]
                      n178 = property on="Senal EMG" class="WFGraph (strict)"("YScale.Maximum"="Y Scale.Range:Maximum") -> ()  [unwired: 2 in, 2 out]
                    }
                    frame 1 {
                    }
                  }
                  n179 = call-poly <vilib>:"Decimate (continuous).vi"("averaging"=TRUE, "decimating factor"=w327, "X"=w328) -> ("Decimated Array"=w324:dbl[])  [unwired: 7 in, 1 out]
                  n180 = Lossy Enqueue Element(queue=w326, element=w324, error in (no error)=w325) -> ()  [unwired: 4 out]
                  n181 = property on="Senal EMG" class="WFGraph (strict)"("YScale.ScaleFit"="Escala automatica Y") -> ()  [unwired: 2 in, 2 out]
                  n182 = property on="Senal EMG" class="WFGraph (strict)"("XScale.ScaleFit"="Escala automatica X") -> ()  [unwired: 2 in, 2 out]
                  n183 = local read "Ganancia"() -> (w321:u16)
                  n184 = event shown="[0] \"Ganancia\": Value Change" {
                    selector: _ -> [_ _]
                    dyn-events: _ -> [_ _]
                    timeout: 10 -> [_ _]
                    tunnel: w321 -> [w342 _]
                    event "Ganancia": Value Change {
                      n185 = event-data() -> ()  [unwired: 1 in, 4 out]
                      n186 = call "Ganancia programable.vi"("MOSI data"=w342) -> ()
                    }
                    event Timeout {
                      n187 = event-data() -> ()  [unwired: 1 in, 3 out]
                    }
                  }
                }
                n188 = VISA Close(VISA resource name=w39, error in (no error)=w38) -> (error out=w40:errorcluster)
                n189 = call <vilib>:"DAQmx Clear Task.vi"("task in"=w97, "error in"=w98) -> ()  [unwired: 13 in, 1 out]
                n190 = Flush Queue(queue=w60) -> ()  [unwired: 1 in, 3 out]
                n191 = call <vilib>:"Simple Error Handler.vi"("error in (no error)"=w40) -> ("error out"=→"error out 2":errorcluster)  [unwired: 4 in, 4 out]
                n192 = VISA Close(VISA resource name=w66, error in (no error)=w68) -> (error out=w69:errorcluster)
                n193 = call <vilib>:"Simple Error Handler.vi"("error in (no error)"=w69) -> ("error out"=→"error out":errorcluster)  [unwired: 4 in, 4 out]
              }
              frame 2 {
                w368 = u16 0 items=["None", "Last Bit", "TermChar", "Break"] ("Serial Settings:End Mode for Writes")
                w367 = u16 2 items=["None", "Last Bit", "TermChar"] ("Serial Settings:End Mode for Reads")
                w381 = u16 0 items=["None", "Last Bit", "TermChar", "Break"] ("Serial Settings:End Mode for Writes")
                w380 = u16 2 items=["None", "Last Bit", "TermChar"] ("Serial Settings:End Mode for Reads")
                # "Close VISA port after program stop. Otherwise this port is blocked."
                # "Close VISA port after program stop. Otherwise this port is blocked."
                # "PwTA command to set temperature limits: PwTA as ASCII characters followed by 45 and 20 degrees in binary code."
                # "Initialize VISA port with correct parameters"
                # "PwTA command to set temperature limits: PwTA as ASCII characters followed by 45 and 20 degrees in binary code."
                # "Initialize VISA port with correct parameters"
                n194 = local read "VISA resource name"() -> (w358:string)
                n195 = call-poly "VISA Configure Serial Port"("VISA resource name"=w358, "timeout (10sec)"=u32 2000, "Enable Termination\nChar (T)"=FALSE ("Enable Termination\nChar (T)"), "baud rate (9600)"=u32 115200, "error in (no error)"="error in (no error) 3") -> ("VISA resource name out"=w363:refnum<visa-resource-name>, "error out"=w365:errorcluster)  [unwired: 9 in]
                n196 = property class="Instr"(reference=w363, error in=w365, "TermChar"=u8 10 ("Message Based Settings:Termination Character"), "ASRL End In"=w367, "ASRL End Out"=w368) -> (reference out=w364:refnum<visa-resource-name>, error out=w366:errorcluster)
                n197 = VISA Set I/O Buffer Size(VISA resource name=w364, error in (no error)=w366) -> (VISA resource name out=w370:refnum<visa-resource-name>, error out=w371:errorcluster)  [unwired: 2 in]
                n198 = VISA Flush I/O Buffer(VISA resource name=w370, error in (no error)=w371) -> (VISA resource name out=w357:refnum<visa-resource-name>, error out=w356:errorcluster)  [unwired: 1 in]
                n199 = case shown="No Error" w356 {
                  tunnel: w356 -> [w403 w437]
                  tunnel: w357 -> [w402 w438]
                  tunnel: [w401 w437] -> w352
                  tunnel: [w400 w438] -> w353
                  frame No Error {
                    w399 = 2 ("length (rest)")
                    # "Initialize Lens Driver"
                    n200 = local read "Calibration"() -> (w390:T3)
                    n201 = for {
                      tunnel: w402 -> [w435]
                      tunnel: [w432] -> w394
                      tunnel: string[] ["Start", "MwCA", "CrMA00", "CrMB00", "CrUA00", "CrUB00", "CrLA00", "CrLB00", "PwTA\u0002Ð\u0001@"] -> [w430] mode=indexing
                      tunnel: [w429] -> w393
                      shift-right: [w433] -> w395
                      shift-left: w390 -> [w434]
                      shift-right: [w431] -> w396
                      shift-left: w403 -> [w436]
                      n202 = call "write read Lens Driver.vi"("VISA resource name"=w435, "command"=w430, "Calibration"=w434, "error in (no error)"=w436) -> ("VISA resource name out"=w432:refnum<visa-resource-name>, "Calibration 2"=w433:T3, "Data"=w429:string, "error out"=w431:errorcluster)  [unwired: 4 in, 4 out]
                    }
                    n203 = String Subset(string=w393, offset (0)=w399, length (rest)=w399) -> (substring=w397:string)
                    n204 = Type Cast(type=u16 0 ("length (rest)"), x=w397) -> (*(type *) &x=w391:u16)
                    n205 = local write "ID"(w391) -> ()
                    n206 = while {
                      tunnel: [w405] -> w401
                      tunnel: [w406] -> w400
                      tunnel: w396 -> [w411]
                      tunnel: w395 -> [w410]
                      tunnel: w394 -> [w409]
                      stop <- w404 stop-if-true
                      # "When Send command is true, Current Ch A is sent to the Lens Driver, in the correct format. If answer exists it is displayed in Data. The update rate of the while loop is 2ms."
                      n207 = Wait Until Next ms Multiple(millisecond multiple=u32 2) -> ()  [unwired: 1 out]
                      n208 = case shown="True" TRUE ("Send command") {
                        tunnel: [w413 w428] -> w405
                        tunnel: w411 -> [w413 w427]
                        tunnel: w410 -> [_ w425]
                        tunnel: w409 -> [w412 w426]
                        tunnel: [w412 w415] -> w406
                        frame False {
                        }
                        frame True {
                          n209 = Multiply(x=200.0, y="Potencia inicial lente derecho") -> (x*y=w423:dbl)
                          n210 = To Word Integer(number=w423) -> (16bit integer=w422:i16)
                          n211 = Type Cast(x=w422) -> (*(type *) &x=w421:string)  [unwired: 1 in]
                          n212 = Concatenate Strings("PwDA", w421) -> (w417:string)
                          n213 = local write "Command to Port"(w417) -> ()
                          n214 = call "write read Lens Driver.vi"("VISA resource name"=w426, "command"=w417, "Calibration"=w425, "error in (no error)"=w427) -> ("VISA resource name out"=w415:refnum<visa-resource-name>, "Calibration 2"=w419:T3, "OK"=w418:bool, "Data"=w416:string, "error out"=w428:errorcluster)  [unwired: 4 in, 3 out]
                          n215 = local write "VISA resource name out"(w415) -> ()
                          n216 = local write "Calibration 2"(w419) -> ()
                          n217 = local write "Data"(w416) -> ()
                          n218 = local write "OK"(w418) -> ()
                          "DPT INICIALES D" <- "Potencia inicial lente derecho"
                        }
                      }
                      n219 = local read "Parar adquisicion"() -> (w404:bool)
                    }
                  }
                  frame Error {
                  }
                }
                n220 = VISA Close(VISA resource name=w353, error in (no error)=w352) -> (error out=w355:errorcluster)
                n221 = call <vilib>:"Simple Error Handler.vi"("error in (no error)"=w355) -> ("error out"=→"error out 3":errorcluster)  [unwired: 4 in, 4 out]
                n222 = local read "VISA resource name 2"() -> (w372:string)
                n223 = call-poly "VISA Configure Serial Port"("VISA resource name"=w372, "timeout (10sec)"=u32 2000, "Enable Termination\nChar (T)"=FALSE ("Enable Termination\nChar (T)"), "baud rate (9600)"=u32 115200, "error in (no error)"="error in (no error) 4") -> ("VISA resource name out"=w376:refnum<visa-resource-name>, "error out"=w378:errorcluster)  [unwired: 9 in]
                n224 = property class="Instr"(reference=w376, error in=w378, "TermChar"=u8 10 ("Message Based Settings:Termination Character"), "ASRL End In"=w380, "ASRL End Out"=w381) -> (reference out=w377:refnum<visa-resource-name>, error out=w379:errorcluster)
                n225 = VISA Set I/O Buffer Size(VISA resource name=w377, error in (no error)=w379) -> (VISA resource name out=w383:refnum<visa-resource-name>, error out=w384:errorcluster)  [unwired: 2 in]
                n226 = VISA Flush I/O Buffer(VISA resource name=w383, error in (no error)=w384) -> (VISA resource name out=w386:refnum<visa-resource-name>, error out=w385:errorcluster)  [unwired: 1 in]
                n227 = case shown="No Error" w385 {
                  tunnel: w385 -> [w452 w486]
                  tunnel: w386 -> [w451 w487]
                  tunnel: [w450 w486] -> w349
                  tunnel: [w449 w487] -> w348
                  frame No Error {
                    w448 = 2 ("length (rest)")
                    # "Initialize Lens Driver"
                    n228 = local read "Calibration"() -> (w439:T3)
                    n229 = for {
                      tunnel: w451 -> [w484]
                      tunnel: [w481] -> w443
                      tunnel: string[] ["Start", "MwCA", "CrMA00", "CrMB00", "CrUA00", "CrUB00", "CrLA00", "CrLB00", "PwTA\u0002Ð\u0001@"] -> [w479] mode=indexing
                      tunnel: [w478] -> w442
                      shift-right: [w482] -> w444
                      shift-left: w439 -> [w483]
                      shift-right: [w480] -> w445
                      shift-left: w452 -> [w485]
                      n230 = call "write read Lens Driver.vi"("VISA resource name"=w484, "command"=w479, "Calibration"=w483, "error in (no error)"=w485) -> ("VISA resource name out"=w481:refnum<visa-resource-name>, "Calibration 2"=w482:T3, "Data"=w478:string, "error out"=w480:errorcluster)  [unwired: 4 in, 4 out]
                    }
                    n231 = String Subset(string=w442, offset (0)=w448, length (rest)=w448) -> (substring=w446:string)
                    n232 = Type Cast(type=u16 0 ("length (rest)"), x=w446) -> (*(type *) &x=w440:u16)
                    n233 = local write "ID"(w440) -> ()
                    n234 = while {
                      tunnel: [w454] -> w450
                      tunnel: [w455] -> w449
                      tunnel: w445 -> [w460]
                      tunnel: w444 -> [w459]
                      tunnel: w443 -> [w458]
                      stop <- w453 stop-if-true
                      # "When Send command is true, Current Ch A is sent to the Lens Driver, in the correct format. If answer exists it is displayed in Data. The update rate of the while loop is 2ms."
                      n235 = Wait Until Next ms Multiple(millisecond multiple=u32 2) -> ()  [unwired: 1 out]
                      n236 = case shown="True" TRUE ("Send command") {
                        tunnel: [w462 w477] -> w454
                        tunnel: w460 -> [w462 w476]
                        tunnel: w459 -> [_ w474]
                        tunnel: w458 -> [w461 w475]
                        tunnel: [w461 w464] -> w455
                        frame False {
                        }
                        frame True {
                          n237 = Multiply(x=200.0, y="Potencia inicial lente izquierdo") -> (x*y=w472:dbl)
                          n238 = To Word Integer(number=w472) -> (16bit integer=w471:i16)
                          n239 = Type Cast(x=w471) -> (*(type *) &x=w470:string)  [unwired: 1 in]
                          n240 = Concatenate Strings("PwDA", w470) -> (w466:string)
                          n241 = local write "Command to Port"(w466) -> ()
                          n242 = call "write read Lens Driver.vi"("VISA resource name"=w475, "command"=w466, "Calibration"=w474, "error in (no error)"=w476) -> ("VISA resource name out"=w464:refnum<visa-resource-name>, "Calibration 2"=w468:T3, "OK"=w467:bool, "Data"=w465:string, "error out"=w477:errorcluster)  [unwired: 4 in, 3 out]
                          n243 = local write "VISA resource name out 2"(w464) -> ()
                          n244 = local write "Calibration 2"(w468) -> ()
                          n245 = local write "Data"(w465) -> ()
                          n246 = local write "OK"(w467) -> ()
                          "DPT INICIALES I" <- "Potencia inicial lente izquierdo"
                        }
                      }
                      n247 = local read "Parar adquisicion"() -> (w453:bool)
                    }
                  }
                  frame Error {
                  }
                }
                n248 = VISA Close(VISA resource name=w348, error in (no error)=w349) -> (error out=w351:errorcluster)
                n249 = call <vilib>:"Simple Error Handler.vi"("error in (no error)"=w351) -> ("error out"=→"error out 4":errorcluster)  [unwired: 4 in, 4 out]
              }
              frame 1 {
                n250 = property on="Waveform length" class="WFChart (strict)"("History Data"=dbl[][] [[0.0]]) -> ()  [unwired: 2 in, 2 out]
                n251 = property on="Potencia optica y distancia" class="WFChart (strict)"("History Data"=dbl[][] [[0.0]]) -> ()  [unwired: 2 in, 2 out]
                n252 = Two Button Dialog(message="Con quien desea realizar los experimentos?", 1:"Nuevo voluntario" ("F button name (\"Cancel\")"), 2:"Voluntario actual" ("T button name (\"OK\")")) -> (T button?=w507:bool)
                n253 = flat-sequence {
                  tunnel: w507 -> [w520]
                  tunnel: [w519] -> w505
                  tunnel: w504 -> [w519]
                  tunnel: [w512] -> w491
                  tunnel: w490 -> [w512]
                  tunnel: [w530] -> w508
                  tunnel: [w532] -> w506
                  tunnel: w505 -> [w532]
                  tunnel: [w531] -> w502
                  tunnel: w501 -> [w531]
                  tunnel: [w529] -> w492
                  tunnel: w491 -> [w529]
                  tunnel: w508 -> [w544]
                  tunnel: w506 -> [w543]
                  tunnel: [w542] -> w503
                  tunnel: w502 -> [w541]
                  tunnel: [w540] -> w499
                  tunnel: [w539] -> w498
                  tunnel: [w538] -> w495
                  tunnel: [w537] -> w493
                  tunnel: w492 -> [w537]
                  tunnel: w499 -> [w596]
                  tunnel: w498 -> [w579]
                  tunnel: [w596] -> w496
                  tunnel: w495 -> [w582]
                  tunnel: [w569] -> w494
                  tunnel: w493 -> [w569]
                  tunnel: [w599] -> w500
                  tunnel: w496 -> [w599]
                  tunnel: w494 -> [w597]
                  frame #0 {
                    # "Se guardan los datos de un nuevo voluntario"
                    n254 = Not(x=w520) -> (.not. x?=w514:bool)
                    n255 = case shown="False" w514 {
                      tunnel: [w523 w528] -> w518
                      tunnel: [w522 w527] -> w517
                      tunnel: [w524 w526] -> w516
                      tunnel: [w521 w525] -> w515
                      frame False {
                        n256 = local read "Enfermedad visual"() -> (w523:string)
                        n257 = local read "Nombre"() -> (w524:string)
                        n258 = local read "Cedula"() -> (w521:string)
                        n259 = local read "Edad"() -> (w522:string)
                      }
                      frame True {
                        n260 = call "Registro voluntario"() -> ("Enfermedad visual"=w528:string, "Edad"=w527:string, "Cedula"=w525:string, "Nombre"=w526:string)  [unwired: 14 in, 2 out]
                      }
                    }
                    "Cedula" <- w515
                    "Nombre" <- w516
                    "Edad" <- w517
                    "Enfermedad visual" <- w518
                    n261 = local write "T button?"(FALSE ("T button?")) -> ()
                  }
                  frame #1 {
                    n262 = Two Button Dialog(message="Qué tipo de experimento desea realizar?", 1:"Nuevo Experimento" ("F button name (\"Cancel\")"), 2:"Experimento existente" ("T button name (\"OK\")")) -> (T button?=w533:bool)
                    n263 = Not(x=w533) -> (.not. x?=w530:bool)
                  }
                  frame #2 {
                    # "A partir de la seleccion del experimento, se obtiene la descripcion correspondiente que será guardada en el archivo"
                    n264 = case shown="False" w544 {
                      tunnel: w543 -> [w546 w564]
                      tunnel: [w546 w563] -> w542
                      tunnel: w541 -> [w548 w562]
                      tunnel: [w548 w561] -> w540
                      tunnel: [w549 w560] -> w539
                      tunnel: [w545 w559] -> w538
                      frame False {
                        n265 = call "Display Message to User"() -> ()  [unwired: 10 in, 2 out]
                        n266 = flat-sequence {
                          tunnel: [w550] -> w547
                          tunnel: w546 -> [w550]
                          tunnel: [w558] -> w549
                          tunnel: w548 -> [w557]
                          tunnel: ["Menu experimentos"] -> _
                          tunnel: w547 -> [w555]
                          tunnel: [w554] -> w545
                          frame #0 {
                            n267 = while {
                              stop <- w551 stop-if-true
                              # "El sistema se queda en el loop hasta que el usuario elija el experimento que desea realizar"
                              n268 = event shown="[0] \"Elegir menu Exp\": Value Change" {
                                selector: _ -> [_ _]
                                dyn-events: _ -> [_ _]
                                timeout: _ -> [_ _]
                                tunnel: [TRUE FALSE] -> w551
                                event "Elegir menu Exp": Value Change {
                                n269 = event-data() -> ()  [unwired: 1 in, 4 out]
                                }
                                event Timeout {
                                n270 = event-data() -> ()  [unwired: 1 in, 3 out]
                                }
                              }
                            }
                          }
                          frame #1 {
                            n271 = Index Array(array=w557, index="Menu experimentos") -> (element=w558:string)
                            n272 = Index Array(array=w555, index="Menu experimentos") -> (element=w554:string)
                          }
                        }
                      }
                      frame True {
                        # "Se añade el nuevo experimento al menu de seleccion de experimentos"
                        # "Se guarda el nuevo experimento en el archivo que los contiene"
                        n273 = call "Nuevo experimento"() -> ("Descripcion"=w560:string, "Nombre"=w559:string)  [unwired: 16 in, 2 out]
                        n274 = Insert Into Array(array=w562, new element=w560) -> (w561:string[])  [unwired: 1 in]
                        n275 = Insert Into Array(array=w564, new element=w559) -> (w563:string[])  [unwired: 1 in]
                        n276 = property on="Menu experimentos" class="Ring (strict)"("Strings []"=w563) -> ()  [unwired: 2 in, 2 out]
                        n277 = Insert Into Array(array=string[] [], new element #1=w559, new element #2=w560) -> (w566:string[])  [unwired: 1 in]
                        n278 = call-poly <vilib>:"Write Delimited Spreadsheet.vi"("file path (dialog if empty)"=path "C:/Users/TGM1603/Documents/LabVIEW Data/Experimentos_realizados", "1D data"=w566, "append to file? (new file:F)"=TRUE) -> ()  [unwired: 11 in, 2 out]
                      }
                    }
                  }
                  frame #3 {
                    # "Se guardan los datos generales del experimento en el archivo de excel"
                    n279 = local read "Frecuencia muestreo"() -> (w571:i32)
                    n280 = local read "factor decimacion"() -> (w578:i32)
                    n281 = local read "Enfermedad visual"() -> (w581:string)
                    n282 = local read "Cedula"() -> (w583:string)
                    n283 = local read "Edad"() -> (w580:string)
                    n284 = local read "Rango voltaje"() -> (w575:i16)
                    n285 = local read "Nombre"() -> (w584:string)
                    n286 = Get Date/Time In Seconds() -> (seconds since 1Jan1904=w595:timestamp)
                    n287 = Path To String(path="Carpeta") -> (string=w591:string)
                    n288 = Format Date/Time String(time format string (%c)="_%d-%m-%y_%H-%M", seconds (now)=w595) -> (date/time string=w593:string)  [unwired: 1 in]
                    n289 = Number To Fractional String(number=w575, precision (6)=i16 0) -> (F-format string=w574:string)  [unwired: 2 in]
                    n290 = Number To Fractional String(number=w578, precision (6)=i16 0) -> (F-format string=w577:string)  [unwired: 2 in]
                    n291 = local read "Cedula"() -> (w587:string)
                    n292 = Number To Fractional String(number=w571, precision (6)=i16 0) -> (F-format string=w572:string)  [unwired: 2 in]
                    n293 = Concatenate Strings(w591, "\\" ("string"), w587, w593, "_" ("string"), w582, ".xlsx" ("string")) -> (w589:string)
                    n294 = String To Path(string=w589) -> (path=w588:path)
                    "path" <- w588
                    n295 = call "MS Office Report"("Path to Save Report"=w588, "Cedula"=w583, "decimacion"=w577, "Edad"=w580, "Enfermedad"=w581, "Exp_nombre"=w582, "Experimento"=w579, "freq"=w572, "Nombre"=w584, "rango"=w574) -> ()  [unwired: 16 in, 2 out]
                  }
                  frame #4 {
                    n296 = while {
                      shift-right: [w601] -> _
                      shift-left: enum16{"Inicio", "Tomar datos", ""}."Inicio" -> [w603]
                      tunnel: w597 -> [w600]
                      stop <- w602 stop-if-true
                      n297 = case shown="\"Tomar datos\"" w603 {
                        tunnel: [w604 w615] -> w601
                        tunnel: w600 -> [_ w610]
                        frame "Inicio", Default {
                          # "Se chequea si el usuario ha presionado el boton de comenzar el experimento. Si no lo ha hecho, se queda en este estado (0).\n Cuando lo presiona, pasa al estado de adquirir datios (1) ."
                          n298 = Select(t=enum16{"Inicio", "Tomar datos", ""}."Tomar datos", s="Iniciar experimento", f=enum16{"Inicio", "Tomar datos", ""}."Inicio") -> (s? t:f=w604:enum16{"Inicio", "Tomar datos", ""})
                        }
                        frame "Tomar datos" {
                          n299 = flat-sequence {
                            tunnel: [w699] -> w614
                            tunnel: [w698] -> w613
                            tunnel: [w697] -> w612
                            tunnel: [w696] -> w611
                            tunnel: w610 -> [w690]
                            tunnel: [w673] -> w609
                            tunnel: [w653] -> w608
                            tunnel: w614 -> [w1020]
                            tunnel: w613 -> [w1019]
                            tunnel: w612 -> [w1018]
                            tunnel: w611 -> [w1017]
                            tunnel: w609 -> [w1014]
                            tunnel: w608 -> [w1015]
                            tunnel: [enum16{"Inicio", "Tomar datos", ""}."Inicio"] -> w615
                            frame #0 {
                              w639 = u16 0 items=["None", "Last Bit", "TermChar", "Break"] ("Serial Settings:End Mode for Writes")
                              w640 = u16 2 items=["None", "Last Bit", "TermChar"] ("Serial Settings:End Mode for Reads")
                              w664 = u16 0 items=["None", "Last Bit", "TermChar", "Break"] ("Serial Settings:End Mode for Writes")
                              w665 = u16 2 items=["None", "Last Bit", "TermChar"] ("Serial Settings:End Mode for Reads")
                              w688 = 100  # max queue size
                              # "Initialize VISA port with correct parameters"
                              # "Initialize VISA port with correct parameters"
                              # "Close VISA port after program stop. Otherwise this port is blocked."
                              # "Se adquiere la señal del circuito de adquisicion, en donde se define la frecuencia de muestreo y el factor de decimacion.\n[1] Se inicializa el canal de adquisicion\n[2] Se ajusta el canal para que lea muestras continuas y apartir de estas prooduzca waveform data.\n[3]  Se obtiene los datos de la señal: la amplitud Y, el tiempo de inicio y el delta t.\n[4] Se decima el vector de amplitud. \n[5] Se usan registros de desplazamiento para concatenenar en un solo vector los datos de la amplitud que se obtienen en cada iteración. \n[6] Se obtiene el ve ctor del tiempo."
                              # "[11] Los vectores de amplitud y tiempo se transforman a formato texto con 4 y 5 cifras significativas respectivamente y se unen para formar un vector de 2 columnas."
                              # "[9] Se ajusta el vector del tiempo para que se muestre un tiempo relativo, es decir, en donde el primer dato sea 0 y en los demas se aumente un dt. \n[10] Se extrae el primer elemento del vector ya que este siempre es 0 y no aporta información"
                              # "[12]"
                              # "[11]"
                              # "[10]"
                              # "[9]"
                              # "[8] Se guarda la fecha/hora en que se inicio el experimento"
                              # "[7] Se usan registros de desplazamiento para concatenar en un solo vector los datos del tiempo que se obtienen en cada iteracion."
                              # "Se define el rango de voltaje de adquisicon"
                              # "[1]"
                              n300 = while {
                                stop <- w735 stop-if-true
                                n301 = local read "Modo de video"() -> (w730:u16)
                                n302 = local read "Frame Rate"() -> (w731:u32)
                                n303 = local read "Carpeta archivo"() -> (w733:string)
                                n304 = local read "Calidad"() -> (w729:u32)
                                n305 = local read "Parar adquisicion"() -> (w734:bool)
                                n306 = call "grabarVideo.vi"("VideoMode"=w730, "Quality"=w729, "Stop (F)"=w734, "Image Logging Path"=w733, "Frame Rate"=w731) -> ("Image Out"=w732:T1, "Stopped"=w735:bool)  [unwired: 20 in, 1 out]
                                n307 = local write "Image Out"(w732) -> ()
                              }
                              n308 = local read "error in (no error)"() -> (w660:errorcluster)
                              n309 = local read "VISA resource name"() -> (w659:string)
                              n310 = local read "VISA resource name 2"() -> (w635:string)
                              n311 = call-poly "VISA Configure Serial Port"("VISA resource name"=w659, "timeout (10sec)"=u32 2000, "Enable Termination\nChar (T)"=FALSE ("Enable Termination\nChar (T)"), "baud rate (9600)"=u32 115200, "error in (no error)"=w660) -> ("VISA resource name out"=w669:refnum<visa-resource-name>, "error out"=w667:errorcluster)  [unwired: 9 in]
                              n312 = call-poly "VISA Configure Serial Port"("VISA resource name"=w635, "timeout (10sec)"=u32 2000, "Enable Termination\nChar (T)"=FALSE ("Enable Termination\nChar (T)"), "baud rate (9600)"=u32 115200, "error in (no error)"="error in (no error) 5") -> ("VISA resource name out"=w644:refnum<visa-resource-name>, "error out"=w642:errorcluster)  [unwired: 9 in]
                              n313 = property class="Instr"(reference=w669, error in=w667, "TermChar"=u8 10 ("Message Based Settings:Termination Character"), "ASRL End In"=w665, "ASRL End Out"=w664) -> (reference out=w668:refnum<visa-resource-name>, error out=w666:errorcluster)
                              n314 = property class="Instr"(reference=w644, error in=w642, "TermChar"=u8 10 ("Message Based Settings:Termination Character"), "ASRL End In"=w640, "ASRL End Out"=w639) -> (reference out=w643:refnum<visa-resource-name>, error out=w641:errorcluster)
                              n315 = VISA Set I/O Buffer Size(VISA resource name=w668, error in (no error)=w666) -> (VISA resource name out=w662:refnum<visa-resource-name>, error out=w661:errorcluster)  [unwired: 2 in]
                              n316 = VISA Set I/O Buffer Size(VISA resource name=w643, error in (no error)=w641) -> (VISA resource name out=w637:refnum<visa-resource-name>, error out=w636:errorcluster)  [unwired: 2 in]
                              n317 = local read "Rango voltaje"() -> (w711:i16)
                              n318 = VISA Flush I/O Buffer(VISA resource name=w662, error in (no error)=w661) -> (VISA resource name out=w658:refnum<visa-resource-name>, error out=w657:errorcluster)  [unwired: 1 in]
                              n319 = VISA Flush I/O Buffer(VISA resource name=w637, error in (no error)=w636) -> (VISA resource name out=w633:refnum<visa-resource-name>, error out=w632:errorcluster)  [unwired: 1 in]
                              n320 = local read "Frecuencia muestreo"() -> (w712:i32)
                              n321 = local read "DAQmx Physical Channel"() -> (w713:tag)
                              n322 = invoke on="Parar adquisicion" class="Bool (strict)" method="Reinit To Default"() -> ()  [unwired: 3 in, 3 out]
                              n323 = Enqueue Element(queue=w690, element=0.0) -> (queue out=w693:refnum<queue>)  [unwired: 2 in, 2 out]
                              n324 = Obtain Queue(max queue size (-1, unlimited)=w688, element data type="Cola tipo 2") -> (queue out=w687:refnum<queue>)  [unwired: 3 in, 2 out]
                              n325 = Multiply(x=-1.0 ("y"), y=w711) -> (x*y=w719:dbl)
                              n326 = call "Analog channel - inicializacion.vi"("maximum value"=w711, "minimum value"=w719, "rate"=w712, "DAQmx Physical Channel"=w713) -> ("error out"=w718:errorcluster, "task out"=w717:refnum<k21>)
                              n327 = local read "tamaño buffer"() -> (w714:i32)
                              n328 = call <vilib>:"DAQmx Start Task.vi"("task/channels in"=w717, "error in"=w718) -> ("task out"=w715:refnum<k21>, "error out"=w716:errorcluster)  [unwired: 12 in]
                              n329 = case shown="No Error" w657 {
                                tunnel: w657 -> [w830 w926]
                                tunnel: w658 -> [w829 w927]
                                tunnel: [w828 w926] -> w685
                                tunnel: [w827 w927] -> w684
                                tunnel: [w815 dbl[] [-1.0]] -> w677
                                tunnel: [w814 dbl[] [-30.0]] -> w625
                                tunnel: [w813 u32[] [0]] -> w655
                                tunnel: [w811 dbl[] [-30.0]] -> w628
                                frame No Error {
                                w826 = 2 ("length (rest)")
                                # "Initialize Lens Driver"
                                n330 = local read "Calibration"() -> (w817:T3)
                                n331 = for {
                                tunnel: w829 -> [w920]
                                tunnel: [w917] -> w821
                                tunnel: string[] ["Start", "MwCA", "CrMA00", "CrMB00", "CrUA00", "CrUB00", "CrLA00", "CrLB00", "PwTA\u0002Ð\u0001@"] -> [w915] mode=indexing
                                tunnel: [w914] -> w820
                                shift-right: [w918] -> w822
                                shift-left: w817 -> [w919]
                                shift-right: [w916] -> w823
                                shift-left: w830 -> [w921]
                                n332 = call "write read Lens Driver.vi"("VISA resource name"=w920, "command"=w915, "Calibration"=w919, "error in (no error)"=w921) -> ("VISA resource name out"=w917:refnum<visa-resource-name>, "Calibration 2"=w918:T3, "Data"=w914:string, "error out"=w916:errorcluster)  [unwired: 4 in, 4 out]
                                }
                                n333 = String Subset(string=w820, offset (0)=w826, length (rest)=w826) -> (substring=w824:string)
                                n334 = Type Cast(type=u16 0 ("length (rest)"), x=w824) -> (*(type *) &x=w818:u16)
                                n335 = local write "ID"(w818) -> ()
                                n336 = while {
                                tunnel: [w848] -> w828
                                tunnel: [w849] -> w827
                                tunnel: w823 -> [w854]
                                tunnel: w822 -> [w853]
                                tunnel: w821 -> [w852]
                                shift-right: [w835] -> w815
                                shift-left: dbl[] [0.0] -> [w836]
                                shift-right: [w843] -> w814
                                shift-left: dbl[] [0.0] -> [w846]
                                shift-right: [w842] -> w813
                                shift-left: u32[] [0] -> [w845]
                                shift-right: [w833] -> w811
                                shift-left: dbl[] [0.0] -> [w832]
                                stop <- w847 stop-if-true
                                # "When Send command is true, Current Ch A is sent to the Lens Driver, in the correct format. If answer exists it is displayed in Data. The update rate of the while loop is 2ms."
                                n337 = Wait Until Next ms Multiple(millisecond multiple=u32 10) -> ()  [unwired: 1 out]
                                n338 = case shown="True" TRUE ("Send command") {
                                tunnel: [w861 w880] -> w848
                                tunnel: w854 -> [w861 w879]
                                tunnel: w853 -> [_ w877]
                                tunnel: w852 -> [w860 w878]
                                tunnel: [w860 w866] -> w849
                                tunnel: [dbl[] [-20.0] w865] -> w843
                                tunnel: w846 -> [_ w864]
                                frame False {
                                }
                                frame True {
                                n339 = local read "Potencia inicial lente derecho"() -> (w862:dbl)
                                n340 = local read "number"() -> (w871:u32)
                                n341 = case shown="2" w871 {
                                tunnel: [w881 w890 w905] -> w863
                                tunnel: w862 -> [w883 w885 w900]
                                tunnel: w862 -> [_ w884 w899]
                                frame 0, Default {
                                n342 = local read "DPT dif."() -> (w882:dbl)
                                n343 = Add(x=w883, y=w882) -> (x+y=w881:dbl)
                                }
                                frame 1 {
                                n344 = local read "DPT dif."() -> (w886:dbl)
                                n345 = Add(x=w885, y=w886) -> (x+y=w887:dbl)
                                n346 = Less Or Equal?(x=w887, y=6.0) -> (x <= y?=w889:bool)
                                n347 = case shown="True" w889 {
                                tunnel: [w892 w895] -> w890
                                tunnel: w884 -> [w891 w894]
                                frame False {
                                n348 = local read "DPT dif."() -> (w893:dbl)
                                n349 = Add(x=w891, y=w893) -> (x+y=w892:dbl)
                                }
                                frame True {
                                n350 = local read "DPT dif."() -> (w896:dbl)
                                n351 = Add(x=w896, y="Incremento") -> (x+y=w897:dbl)
                                n352 = local write "DPT dif."(w897) -> ()
                                n353 = Add(x=w894, y=w897) -> (x+y=w895:dbl)
                                }
                                }
                                }
                                frame 2 {
                                n354 = local read "DPT dif."() -> (w904:dbl)
                                n355 = Add(x=w904, y=w900) -> (x+y=w901:dbl)
                                n356 = Greater Or Equal?(x=w901, y=-6.0) -> (x >= y?=w902:bool)
                                n357 = case shown="True" w902 {
                                tunnel: [w907 w911] -> w905
                                tunnel: w899 -> [w906 w910]
                                frame False {
                                n358 = local read "DPT dif."() -> (w908:dbl)
                                n359 = Add(x=w906, y=w908) -> (x+y=w907:dbl)
                                }
                                frame True {
                                n360 = local read "DPT dif."() -> (w913:dbl)
                                n361 = local read "Incremento"() -> (w909:dbl)
                                n362 = Subtract(x=w913, y=w909) -> (x-y=w912:dbl)
                                n363 = local write "DPT dif."(w912) -> ()
                                n364 = Add(x=w910, y=w912) -> (x+y=w911:dbl)
                                }
                                }
                                }
                                }
                                "Potencia derecho" <- w863
                                n365 = Multiply(x=200.0, y=w863) -> (x*y=w875:dbl)
                                n366 = To Word Integer(number=w875) -> (16bit integer=w874:i16)
                                n367 = Type Cast(x=w874) -> (*(type *) &x=w873:string)  [unwired: 1 in]
                                n368 = Concatenate Strings("PwDA", w873) -> (w868:string)
                                n369 = local write "Command to Port"(w868) -> ()
                                n370 = call "write read Lens Driver.vi"("VISA resource name"=w878, "command"=w868, "Calibration"=w877, "error in (no error)"=w879) -> ("VISA resource name out"=w866:refnum<visa-resource-name>, "Calibration 2"=w870:T3, "OK"=w869:bool, "Data"=w867:string, "error out"=w880:errorcluster)  [unwired: 4 in, 3 out]
                                n371 = local write "VISA resource name out"(w866) -> ()
                                n372 = local write "Calibration 2"(w870) -> ()
                                n373 = local write "Data"(w867) -> ()
                                n374 = local write "OK"(w869) -> ()
                                n375 = Build Array (concatenate)(w864, w863) -> (w865:dbl[])
                                }
                                }
                                n376 = local read "Parar adquisicion"() -> (w847:bool)
                                n377 = local read "Potencia izquierdo"() -> (w831:dbl)
                                n378 = local read "Distancia"() -> (w844:u32)
                                n379 = property on="Potencia optica y distancia" class="WFChart (strict)"("YScale.ScaleFit"="Auto scale Y") -> ()  [unwired: 2 in, 2 out]
                                n380 = Get Date/Time In Seconds() -> (seconds since 1Jan1904=w837:timestamp)
                                n381 = To Double Precision Float(number=w837) -> (double precision float=w834:dbl)
                                n382 = property on="Potencia optica y distancia" class="WFChart (strict)"("XScale.ScaleFit"="Auto scale X") -> ()  [unwired: 2 in, 2 out]
                                n383 = Build Array (concatenate)(w836, w834) -> (w835:dbl[])
                                n384 = case shown="0, Default" "Auto scale Y" {
                                frame 0, Default {
                                n385 = property on="Potencia optica y distancia" class="WFChart (strict)"("YScale.Maximum"="Escala Y max") -> ()  [unwired: 2 in, 2 out]
                                n386 = property on="Potencia optica y distancia" class="WFChart (strict)"("YScale.Minimum"="Escala Y min") -> ()  [unwired: 2 in, 2 out]
                                }
                                frame 1 {
                                }
                                }
                                n387 = Build Array (concatenate)(w832, w831) -> (w833:dbl[])
                                n388 = Build Array (concatenate)(w845, w844) -> (w842:u32[])
                                n389 = case shown="0, Default" "Auto scale X" {
                                frame 0, Default {
                                n390 = property on="Potencia optica y distancia" class="WFChart (strict)"("XScale.Maximum"="Escala X max") -> ()  [unwired: 2 in, 2 out]
                                n391 = property on="Potencia optica y distancia" class="WFChart (strict)"("XScale.Minimum"="Escala X min") -> ()  [unwired: 2 in, 2 out]
                                }
                                frame 1 {
                                }
                                }
                                n392 = Build Array(w843, w842) -> (w841:dbl[][])
                                n393 = Transpose 2D Array(2D array=w841) -> (transposed array=→"Potencia optica y distancia":dbl[][])
                                }
                                }
                                frame Error {
                                }
                              }
                              n394 = case shown="No Error" w632 {
                                tunnel: w632 -> [w750 w807]
                                tunnel: w633 -> [w749 w808]
                                tunnel: [w748 w807] -> w618
                                tunnel: [w747 w808] -> w619
                                tunnel: [w736 dbl[] [-30.0]] -> _
                                frame No Error {
                                w746 = 2 ("length (rest)")
                                # "Initialize Lens Driver"
                                n395 = local read "Calibration"() -> (w737:T3)
                                n396 = for {
                                tunnel: w749 -> [w804]
                                tunnel: [w801] -> w741
                                tunnel: string[] ["Start", "MwCA", "CrMA00", "CrMB00", "CrUA00", "CrUB00", "CrLA00", "CrLB00", "PwTA\u0002Ð\u0001@"] -> [w799] mode=indexing
                                tunnel: [w798] -> w740
                                shift-right: [w802] -> w742
                                shift-left: w737 -> [w803]
                                shift-right: [w800] -> w743
                                shift-left: w750 -> [w805]
                                n397 = call "write read Lens Driver.vi"("VISA resource name"=w804, "command"=w799, "Calibration"=w803, "error in (no error)"=w805) -> ("VISA resource name out"=w801:refnum<visa-resource-name>, "Calibration 2"=w802:T3, "Data"=w798:string, "error out"=w800:errorcluster)  [unwired: 4 in, 4 out]
                                }
                                n398 = String Subset(string=w740, offset (0)=w746, length (rest)=w746) -> (substring=w744:string)
                                n399 = Type Cast(type=u16 0 ("length (rest)"), x=w744) -> (*(type *) &x=w738:u16)
                                n400 = local write "ID"(w738) -> ()
                                n401 = while {
                                tunnel: [w755] -> w748
                                tunnel: [w756] -> w747
                                tunnel: w743 -> [w761]
                                tunnel: w742 -> [w760]
                                tunnel: w741 -> [w759]
                                shift-right: [w752] -> w736
                                shift-left: _ -> [w753]
                                stop <- w754 stop-if-true
                                # "When Send command is true, Current Ch A is sent to the Lens Driver, in the correct format. If answer exists it is displayed in Data. The update rate of the while loop is 2ms."
                                n402 = Wait Until Next ms Multiple(millisecond multiple=u32 10) -> ()  [unwired: 1 out]
                                n403 = case shown="True" TRUE ("Send command") {
                                tunnel: [w767 w790] -> w755
                                tunnel: w761 -> [w767 w789]
                                tunnel: w760 -> [_ w787]
                                tunnel: w759 -> [w766 w788]
                                tunnel: [w766 w777] -> w756
                                tunnel: [dbl[] [-20.0] w776] -> w752
                                tunnel: w753 -> [_ w775]
                                frame False {
                                }
                                frame True {
                                n404 = local read "Potencia inicial lente izquierdo"() -> (w774:dbl)
                                n405 = local read "DPT dif."() -> (w773:dbl)
                                n406 = Add(x=w773, y=w774) -> (x+y=w769:dbl)
                                n407 = Absolute Value(x=w769) -> (abs(x)=w771:dbl)
                                n408 = Greater Or Equal?(x=6.0, y=w771) -> (x >= y?=w770:bool)
                                n409 = case shown="False" w770 {
                                tunnel: w769 -> [w793 w797]
                                tunnel: [w791 w797] -> w768
                                frame False {
                                n410 = Greater Or Equal?(x=u16 0, y=w793) -> (x >= y?=w794:bool)
                                n411 = case shown="False" w794 {
                                tunnel: [i16 6 ("x") i16 -6 ("x")] -> w791
                                frame False {
                                }
                                frame True {
                                }
                                }
                                }
                                frame True {
                                }
                                }
                                "Potencia izquierdo" <- w768
                                n412 = Multiply(x=200.0, y=w768) -> (x*y=w785:dbl)
                                n413 = To Word Integer(number=w785) -> (16bit integer=w784:i16)
                                n414 = Type Cast(x=w784) -> (*(type *) &x=w783:string)  [unwired: 1 in]
                                n415 = Concatenate Strings("PwDA", w783) -> (w779:string)
                                n416 = local write "Command to Port"(w779) -> ()
                                n417 = call "write read Lens Driver.vi"("VISA resource name"=w788, "command"=w779, "Calibration"=w787, "error in (no error)"=w789) -> ("VISA resource name out"=w777:refnum<visa-resource-name>, "Calibration 2"=w781:T3, "OK"=w780:bool, "Data"=w778:string, "error out"=w790:errorcluster)  [unwired: 4 in, 3 out]
                                n418 = local write "VISA resource name 2"(w777) -> ()
                                n419 = local write "Calibration 2"(w781) -> ()
                                n420 = local write "Data"(w778) -> ()
                                n421 = local write "OK"(w780) -> ()
                                n422 = Build Array (concatenate)(w775, w768) -> (w776:dbl[])
                                }
                                }
                                n423 = local read "Parar adquisicion"() -> (w754:bool)
                                n424 = event shown="[0] \"Restablecer Iniciales\": Value Change" {
                                selector: _ -> [_ _]
                                dyn-events: _ -> [_ _]
                                timeout: 100 -> [_ _]
                                event "Restablecer Iniciales": Value Change {
                                n425 = event-data() -> ()  [unwired: 1 in, 3 out]
                                n426 = local read "Potencia inicial lente izquierdo"() -> (w762:dbl)
                                n427 = local read "Potencia inicial lente derecho"() -> (w763:dbl)
                                n428 = local write "Potencia izquierdo"(w762) -> ()
                                n429 = local write "Potencia derecho"(w763) -> ()
                                n430 = local write "DPT dif."(0.0 ("DPT dif.")) -> ()
                                }
                                event Timeout {
                                n431 = event-data() -> ()  [unwired: 1 in, 3 out]
                                }
                                }
                                }
                                }
                                frame Error {
                                }
                              }
                              n432 = while {
                                tunnel: w693 -> [w959]
                                shift-right: [w961] -> _
                                shift-left: dbl[] [0.0] -> [w967]
                                shift-right: [w960] -> _
                                shift-left: u32[] [0] -> [w962]
                                tunnel: [w959] -> w691
                                tunnel: w687 -> [w951]
                                stop <- w950 stop-if-true
                                n433 = local read "WL"() -> (w958:dbl)
                                n434 = local read "Parar adquisicion"() -> (w950:bool)
                                n435 = local read "Limite superior WL"() -> (w955:dbl)
                                n436 = call "waveform_length.vi"("WL"=w958, "Cola WL"=w959, "Datos entrada"=w951) -> ("WL 2"=w966:dbl)
                                n437 = local read "Limite inferior WL"() -> (w957:dbl)
                                n438 = local write "WL"(w966) -> ()
                                n439 = Build Array (concatenate)(w967, w966) -> (w961:dbl[])
                                n440 = In Range and Coerce(upper limit=w955, x=w966, lower limit=w957) -> (In Range?=w964:bool)  [unwired: 1 out]
                                n441 = Greater?(x=w966, y=w955) -> (0:w965:bool)
                                n442 = local read "Escala autom. X"() -> (w952:u8)
                                n443 = local read "Escala autom. Y"() -> (w953:u8)
                                n444 = Build Array(w965, w964) -> (w963:bool[])
                                n445 = Boolean Array To Number(Boolean array=w963) -> (number=w956:u32)
                                n446 = local write "number"(w956) -> ()
                                n447 = Build Array (concatenate)(w962, w956) -> (w960:u32[])
                                n448 = Build Array(w961, w960) -> (w954:dbl[][])
                                n449 = Transpose 2D Array(2D array=w954) -> (transposed array=w949:dbl[][])
                                n450 = local write "Waveform length"(w949) -> ()
                                n451 = property on="Waveform length" class="WFChart (strict)"("XScale.ScaleFit"=w952) -> ()  [unwired: 2 in, 2 out]
                                n452 = property on="Waveform length" class="WFChart (strict)"("YScale.ScaleFit"=w953) -> ()  [unwired: 2 in, 2 out]
                                n453 = case shown="0, Default" w953 {
                                frame 0, Default {
                                n454 = local read "Maximo escala Y"() -> (w971:dbl)
                                n455 = local read "Minimo escala Y"() -> (w970:dbl)
                                n456 = property on="Waveform length" class="WFChart (strict)"("YScale.Maximum"=w971) -> ()  [unwired: 2 in, 2 out]
                                n457 = property on="Waveform length" class="WFChart (strict)"("YScale.Minimum"=w970) -> ()  [unwired: 2 in, 2 out]
                                }
                                frame 1 {
                                }
                                }
                                n458 = case shown="0, Default" w952 {
                                frame 0, Default {
                                n459 = local read "Maximo escala X"() -> (w968:dbl)
                                n460 = local read "Minimo escala X"() -> (w969:dbl)
                                n461 = property on="Waveform length" class="WFChart (strict)"("XScale.Maximum"=w968) -> ()  [unwired: 2 in, 2 out]
                                n462 = property on="Waveform length" class="WFChart (strict)"("XScale.Minimum"=w969) -> ()  [unwired: 2 in, 2 out]
                                }
                                frame 1 {
                                }
                                }
                              }
                              n463 = while {
                                tunnel: w715 -> [w1004]
                                tunnel: w714 -> [w1001]
                                tunnel: [w1002] -> w701
                                shift-right: [w999] -> w700
                                shift-left: w716 -> [w1003]
                                tunnel: [w994] -> w728
                                shift-right: [w993] -> w698
                                shift-left: _ -> [w992]
                                shift-right: [w983] -> w703
                                shift-left: dbl[] [0.0] -> [w988]
                                shift-right: [w984] -> w708
                                shift-left: dbl[] [0.0] -> [w985]
                                tunnel: w687 -> [w976]
                                i -> [w995]
                                stop <- w998 stop-if-true
                                w997 = 10.0  # timeout (s)
                                # "El sistema se queda en el loop hasta que el usuario decida iniciar el experimento"
                                # "[7]"
                                # "[6]"
                                # "[5]"
                                # "[4]"
                                # "[3]"
                                # "[2]"
                                n464 = local read "Escala automatica X"() -> (w974:u8)
                                n465 = local read "Escala automatica Y"() -> (w973:u8)
                                n466 = property on="Senal EMG" class="WFGraph (strict)"("XScale.ScaleFit"=w974) -> ()  [unwired: 2 in, 2 out]
                                n467 = case shown="0, Default" w974 {
                                frame 0, Default {
                                n468 = local read "X Scale.Range:Increment"() -> (w1007:dbl)
                                n469 = local read "X Scale.Range:Maximum"() -> (w1009:dbl)
                                n470 = local read "X Scale.Range:Minimum"() -> (w1008:dbl)
                                n471 = property on="Senal EMG" class="WFGraph (strict)"("XScale.Increment"=w1007) -> ()  [unwired: 2 in, 2 out]
                                n472 = property on="Senal EMG" class="WFGraph (strict)"("XScale.Minimum"=w1008) -> ()  [unwired: 2 in, 2 out]
                                n473 = property on="Senal EMG" class="WFGraph (strict)"("XScale.Maximum"=w1009) -> ()  [unwired: 2 in, 2 out]
                                }
                                frame 1 {
                                }
                                }
                                n474 = local read "Parar adquisicion"() -> (w979:bool)
                                n475 = call-poly <vilib>:"DAQmx Read.vi"("task/channels in"=w1004, "number of samples per channel"=w1001, "timeout"=w997, "error in"=w1003) -> ("task out"=w1002:refnum<k21>, "data"=w989:waveform(dbl)[], "error out"=w999:errorcluster)  [unwired: 9 in]
                                n476 = Unbundle By Name(w999) -> ("status"=w1000:bool)
                                n477 = Or(x=w1000, y=w979) -> (x .or. y?=w998:bool)
                                n478 = property on="Senal EMG" class="WFGraph (strict)"("YScale.ScaleFit"=w973) -> ()  [unwired: 2 in, 2 out]
                                n479 = local write "Senal EMG"(w989) -> ()
                                n480 = case shown="0, Default" w973 {
                                frame 0, Default {
                                n481 = local read "Y Scale.Range:Maximum"() -> (w1006:dbl)
                                n482 = local read "Y Scale.Range:Minimum"() -> (w1005:dbl)
                                n483 = property on="Senal EMG" class="WFGraph (strict)"("YScale.Minimum"=w1005) -> ()  [unwired: 2 in, 2 out]
                                n484 = property on="Senal EMG" class="WFGraph (strict)"("YScale.Maximum"=w1006) -> ()  [unwired: 2 in, 2 out]
                                }
                                frame 1 {
                                }
                                }
                                n485 = call-poly <vilib>:"Index Waveform Array.vi"("index"=0, "waveform array"=w989) -> ("waveform"=w987:waveform(dbl))  [unwired: 8 in, 1 out]
                                n486 = Unbundle By Name(w987) -> ("Y"=w977:dbl[], "t0"=w994:timestamp)  [unwired: 1 out]
                                n487 = call-poly <vilib>:"Decimate (continuous).vi"("averaging"=TRUE, "decimating factor"="factor decimacion", "X"=w977) -> ("Decimated Array"=w972:dbl[])  [unwired: 7 in, 1 out]
                                n488 = Lossy Enqueue Element(queue=w976, element=w972) -> ()  [unwired: 1 in, 4 out]
                                n489 = Build Array (concatenate)(w988, w972) -> (w983:dbl[])
                                n490 = case shown="0, Default" w995 {
                                tunnel: w994 -> [_ w1013]
                                tunnel: [w1011 w1012] -> w993
                                tunnel: w992 -> [w1011 _]
                                frame 0, Default {
                                }
                                frame 1 {
                                # "[8]"
                                n491 = Format Date/Time String(seconds (now)=w1013) -> (date/time string=w1012:string)  [unwired: 2 in]
                                }
                                }
                                n492 = local read "factor decimacion"() -> (w980:i32)
                                n493 = call-poly <vilib>:"Get Waveform Time Array.vi"("waveform in"=w987) -> ("X array"=w986:timestamp[])  [unwired: 9 in, 1 out]
                                n494 = event shown="[0] \"Ganancia\": Value Change" {
                                selector: _ -> [_ _]
                                dyn-events: _ -> [_ _]
                                timeout: 1 -> [_ _]
                                tunnel: "Ganancia" -> [w1010 _]
                                event "Ganancia": Value Change {
                                n495 = event-data() -> ()  [unwired: 1 in, 4 out]
                                n496 = call "Ganancia programable.vi"("MOSI data"=w1010) -> ()
                                }
                                event Timeout {
                                n497 = event-data() -> ()  [unwired: 1 in, 3 out]
                                }
                                }
                                n498 = To Double Precision Float(number=w986) -> (double precision float=w982:dbl[])
                                n499 = call-poly <vilib>:"Decimate (single shot).vi"("decimating factor"=w980, "X"=w982) -> ("Decimated Array"=w981:dbl[])  [unwired: 8 in, 1 out]
                                n500 = Build Array (concatenate)(w985, w981) -> (w984:dbl[])
                              }
                              n501 = call <vilib>:"DAQmx Clear Task.vi"("task in"=w701, "error in"=w700) -> ()  [unwired: 13 in, 1 out]
                              n502 = Index Array(array=w708, index=1) -> (element=w707:dbl)
                              n503 = Flush Queue(queue=w691) -> ()  [unwired: 1 in, 3 out]
                              n504 = Subtract(x=w708, y=w707) -> (x-y=w705:dbl[])
                              n505 = Delete From Array(array=w703, index=0) -> (array with subset deleted=w723:dbl[])  [unwired: 1 in, 1 out]
                              n506 = while {
                                shift-right: [w928] -> _
                                shift-left: _ -> [w929]
                                stop <- w933 stop-if-true
                                # "Este bloque adquiere la distancia"
                                n507 = call "meididor de distancia archivo adicional.vi"() -> ("error out"=w936:errorcluster, "task out"=w937:refnum<k21>)  [unwired: 10 in]
                                n508 = call "DAQ Assistant2"("timeout (s)"=0.05) -> ("data"=w946:dynamicdata, "error out"=w934:errorcluster)  [unwired: 16 in, 1 out]
                                n509 = call <vilib>:"DAQmx Start Task.vi"("task/channels in"=w937, "error in"=w936) -> ("task out"=w940:refnum<k21>, "error out"=w941:errorcluster)  [unwired: 12 in]
                                n510 = call <vilib>:"DAQmx Is Task Done.vi"("task/channels in"=w940, "error in"=w941) -> ("task out"=w938:refnum<k21>, "error out"=w939:errorcluster)  [unwired: 11 in, 1 out]
                                n511 = Wait (ms)(milliseconds to wait=u32 200) -> ()  [unwired: 1 out]
                                n512 = call <vilib>:"Clear Errors.vi"("error in (no error)"=w934) -> ()  [unwired: 5 in, 2 out]
                                n513 = local read "Parar adquisicion"() -> (w933:bool)
                                n514 = call <vilib>:"DAQmx Clear Task.vi"("task in"=w938, "error in"=w939) -> ()  [unwired: 13 in, 1 out]
                                n515 = Multiply(x=1000000.0, y=w946) -> (x*y=w944:dynamicdata)
                                n516 = Divide(x=w944, y=58.0) -> (x/y=w930:dynamicdata)
                                n517 = Equal?(x=w930, y=0.0) -> (x = y?=w932:dynamicdata)
                                n518 = case shown="True" w932 {
                                tunnel: [w947 w948] -> w928
                                tunnel: w930 -> [w947 _]
                                tunnel: w929 -> [_ w948]
                                frame False {
                                }
                                frame True {
                                }
                                }
                                n519 = local write "Distancia"(w928) -> ()
                              }
                              n520 = Delete From Array(array=w705, index=0) -> (array with subset deleted=w722:dbl[])  [unwired: 1 in, 1 out]
                              n521 = local read "path"() -> (w699:path)
                              n522 = Format Date/Time String(seconds (now)=w728) -> (date/time string=w697:string)  [unwired: 2 in]
                              n523 = Number To Fractional String(use system decimal point (T)=FALSE, number=w723, precision (6)=i16 4) -> (F-format string=w651:string[])  [unwired: 1 in]
                              n524 = Number To Fractional String(use system decimal point (T)=FALSE, number=w722, precision (6)=i16 5) -> (F-format string=w652:string[])  [unwired: 1 in]
                              n525 = Build Array(w652, w651) -> (w721:string[][])
                              n526 = Transpose 2D Array(2D array=w721) -> (transposed array=w696:string[][])
                              n527 = Delete From Array(array=w625, index=0) -> (array with subset deleted=w624:dbl[])  [unwired: 1 in, 1 out]
                              n528 = Delete From Array(array=w655, index=0) -> (array with subset deleted=w621:u32[])  [unwired: 1 in, 1 out]
                              n529 = Index Array(array=w677, index=1) -> (element=w682:dbl)
                              n530 = VISA Close(VISA resource name=w619, error in (no error)=w618) -> (error out=w617:errorcluster)
                              n531 = Delete From Array(array=w628, index=0) -> (array with subset deleted=w627:dbl[])  [unwired: 1 in, 1 out]
                              n532 = Subtract(x=w677, y=w682) -> (x-y=w676:dbl[])
                              n533 = Number To Fractional String(use system decimal point (T)=FALSE, number=w624, precision (6)=i16 2) -> (F-format string=w648:string[])  [unwired: 1 in]
                              n534 = VISA Close(VISA resource name=w684, error in (no error)=w685) -> (error out=w686:errorcluster)
                              n535 = call <vilib>:"Simple Error Handler.vi"("error in (no error)"=w617) -> ("error out"=w616:errorcluster)  [unwired: 4 in, 4 out]
                              n536 = Number To Fractional String(number=w621, precision (6)=i16 0) -> (F-format string=w649:string[])  [unwired: 2 in]
                              n537 = Delete From Array(array=w676, index=0) -> (array with subset deleted=w681:dbl[])  [unwired: 1 in, 1 out]
                              n538 = call <vilib>:"Simple Error Handler.vi"("error in (no error)"=w686) -> ("error out"=w683:errorcluster)  [unwired: 4 in, 4 out]
                              n539 = Number To Fractional String(use system decimal point (T)=FALSE, number=w627, precision (6)=i16 2) -> (F-format string=w629:string[])  [unwired: 1 in]
                              n540 = local write "error out"(w616) -> ()
                              n541 = local write "error out"(w683) -> ()
                              n542 = Number To Fractional String(use system decimal point (T)=FALSE, number=w681, precision (6)=i16 5) -> (F-format string=w650:string[])  [unwired: 1 in]
                              n543 = Build Array(w652, w651, w650, w649, w648, w629) -> (w622:string[][])
                              n544 = Transpose 2D Array(2D array=w622) -> (transposed array=w653:string[][])
                              n545 = Build Array(w650, w649, w648, w629) -> (w673:string[][])
                            }
                            frame #1 {
                              # "[12] Se invoca la funcion de escribir en un archivo de excel para guadar los datos."
                              n546 = Transpose 2D Array(2D array=w1014) -> (transposed array=w1016:string[][])
                              n547 = call <vilib>:"Three Button Dialog.vi"("Right Button Text (\"Cancel\")"="Señal EMG, potencia optica y distancia" ("Right Button Text (\"Cancel\")"), "Center Button Text (\"No\")"="Potencia optica y distancia" ("Center Button Text (\"No\")"), "Left Button Text (\"Yes\")"="Señal EMG" ("Left Button Text (\"Yes\")"), "message"="Elija que datos desea guardar") -> ("Which Button?"=w1021:T4)  [unwired: 7 in]
                              n548 = case shown="\"Right Button\"" w1021 {
                                tunnel: w1020 -> [w1030 w1035 w1038]
                                tunnel: w1019 -> [w1029 w1034 w1039]
                                tunnel: w1018 -> [w1028 w1033 w1040]
                                tunnel: w1017 -> [w1027 _ _]
                                tunnel: w1016 -> [_ w1032 _]
                                tunnel: w1015 -> [_ _ w1036]
                                frame "Left Button", Default {
                                n549 = call "Guardar datos de Amplitud y Tiempo.vi"("path"=w1030, "Hora inicio"=w1029, "Hora fin"=w1028, "Datos experimento"=w1027, "column headers"=string[] ["Tiempo(s)", "Amplitud(V)"]) -> ()  [unwired: 1 in]
                                }
                                frame "Center Button" {
                                n550 = call "Guardar datos de Amplitud y Tiempo.vi"("path"=w1035, "Hora inicio"=w1034, "Hora fin"=w1033, "Datos experimento"=w1032, "column headers"=string[] ["Tiempo(s)", "Distancia (cm)", "Potencia Optica derecho", "Potencia optica izquierdo"]) -> ()  [unwired: 1 in]
                                }
                                frame "Right Button" {
                                n551 = call "Guardar datos de Amplitud y Tiempo.vi"("path"=w1038, "Hora inicio"=w1039, "Hora fin"=w1040, "Datos experimento"=w1036, "column headers"=string[] ["Tiempo EMG(s)", "Amplitud(V)", "Tiempo DPT(s)", "Distancia (cm)", "Potencia optica derecho", "Potencia optica izquierdo"]) -> ()  [unwired: 1 in]
                                }
                              }
                            }
                            frame #2 {
                              # "Si el usuario desea repetir el experimento se vuelve al estado inicio en donde se espera que comience el experimento. De lo contrario se sale del loop y vuelve al menu principal."
                              n552 = Two Button Dialog(message="¿Desea repetir el experimento?", 1:"No" ("F button name (\"Cancel\")"), 2:"Si" ("T button name (\"OK\")")) -> (T button?=w1043:bool)
                              n553 = Not(x=w1043) -> (.not. x?=→"T button?":bool)
                            }
                          }
                        }
                      }
                      n554 = local read "T button?"() -> (w602:bool)
                    }
                  }
                }
                n555 = Wait (ms)(milliseconds to wait=u32 5000) -> ()  [unwired: 1 out]
              }
            }
          }
          event Timeout {
            n556 = event-data() -> ()  [unwired: 1 in, 3 out]
          }
        }
      }
    }
  }
